vi "TSCAN_UDS.vi"(10 "Data":T3={"Communication message"={"Sender"="", "receiver"="", "message"="", "data"=variant}, "Data"={"Config_parameter"={"Bus_Type"=0, "Channel"=1, "Channels used"=1, "DLL_PATH"=path "", "Read message type"=1, "REC_Channel"=0}, "Send_parameter"={"SendData"=[0, 0, 0, 0, 0, 0, 0, 0, 0, 0, 0, 0, 0, 0, 0, 0, 0, 0, 0, 0, 0, 0, 0, 0, 0, 0, 0, 0, 0, 0, 0, 0, 0, 0, 0, 0, 0, 0, 0, 0, 0, 0, 0, 0, 0, 0, 0, 0, 0, 0, 0, 0, 0, 0, 0, 0, 0, 0, 0, 0, 0, 0, 0, 0, 0, 0, 0, 0, 0, 0, 0, 0, 0, 0, 0], "Data Length"=15, "ID"=0, "Frame Format"=0, "Frame Type"=0, "BRS"=enum."Close", "FD Frame"=0, "async&sync"=enum."async", "Timeout"=0}, "DBC_Ctr"={"DBC Path"=path "", "DBC loading channel"=0, "DatabaseId"=0, "DBMessages"=[], "DBSignals"=[]}, "CAN_Config_Array"=[], "CANFD_Config_Array"=[], "CAN_Config_Regs_Array"=[], "CANFD_Config_Regs_Array"=[], "Blf_Log"={"Blf_Log_PATH"=path ""}, "UDS"={"UDS Control"={"UDS Channel Index"=0, "Request ID"=1992, "Response ID"=2015, "Request ID (Func)"=1, "Session Mode"=1, "Reset Mode"=255, "DTC Mask"=0, "GropOfDTC"=0, "Seed Level"=2, "Seed"=[], "Key Level"=0, "Key"=[], "Read Identifier"=0, "UDS Read Data"=[], "ASCII Data"="", "Write Identifier"=0, "UDS Wrtie Data"=[], "IO Control Identifier"=1, "UDS IOControl Data"=[], "IO Control Mode"=0, "UDS IOControl Read Data"=[], "Routine Control Identifier"=0, "UDS RoutineControl Data"=[], "UDS RoutineControl Read Data"=[], "Routine Control Mode"=1, "SupportFDCAN"=TRUE, "time config"={"p2_timeout"=0, "p2_extended"=0, "s3_servertime"=0, "s3_clienttime"=0}, "ServiceLayer"={"FilledByte"=0, "STMin"=10, "BlockSize"=10, "FCDelay"=10, "MaxLength"=4095}, "Request"=[], "Respond"=[]}, "DiagModuleIndex"=1984}}, "CAN_Buffer"=[], "CANFD_Buffer"=[], "error in"={"status"=FALSE, "code"=0, "source"=""}, "CAN_Period_Datas"=[], "CANFD_period_Datas"=[], "CAN_Filtering_Datas"=[], "CANFD_Filtering_Datas"=[], "AsynCall?"=FALSE} {"Data"."UDS"."UDS Control"."Respond" format="%.0x"; "Data"."UDS"."UDS Control"."Request" format="%.0x"; "Data"."UDS"."UDS Control"."ServiceLayer"."FilledByte" format="%.0x"; "Data"."UDS"."UDS Control"."GropOfDTC" format="%.0x"; "Data"."UDS"."UDS Control"."DTC Mask" format="%.0x"; "Data"."UDS"."UDS Control"."UDS RoutineControl Read Data" format="%.0x"; "Data"."UDS"."UDS Control"."UDS RoutineControl Data" format="%.0x"; "Data"."UDS"."UDS Control"."Routine Control Identifier" format="%.0x"; "Data"."UDS"."UDS Control"."UDS IOControl Read Data" format="%.0x"; "Data"."UDS"."UDS Control"."UDS IOControl Data" format="%.0x"; "Data"."UDS"."UDS Control"."IO Control Identifier" format="%.0x"; "Data"."UDS"."UDS Control"."UDS Wrtie Data" format="%.0x"; "Data"."UDS"."UDS Control"."UDS Read Data" format="%.0x"; "Data"."UDS"."UDS Control"."Write Identifier" format="%.0x"; "Data"."UDS"."UDS Control"."Read Identifier" format="%.0x"; "Data"."UDS"."UDS Control"."Key" format="%.0x"; "Data"."UDS"."UDS Control"."Seed" format="%.0x"; "Data"."UDS"."UDS Control"."Request ID (Func)" format="%.0x"; "Data"."UDS"."UDS Control"."Response ID" format="%.0x"; "Data"."UDS"."UDS Control"."Request ID" format="%.0x"; "Data"."UDS"."UDS Control"."Session Mode" items=["DefaultSession"=1, "ProgrammingSession"=2, "ExtendedDiagnosticSession"=3]; "Data"."UDS"."UDS Control"."Reset Mode" items=["HardReset"=1, "keyOffOnReset"=2, "SoftReset"=3]; "Data"."UDS"."UDS Control"."IO Control Mode" items=["ReturnControlToECU", "ResetToDefault", "FreezeCurrentState", "ShortTermAdjustment"]; "Data"."UDS"."UDS Control"."Routine Control Mode" items=["Start routine"=1, "Stop routine"=2, "Request routine results"=3]; "Data"."CAN_Config_Regs_Array"."CAN configuration"."AAppChannel" items=["CHN1", "CHN2", "CHN3", "CHN4", "CHN5", "CHN6", "CHN7", "CHN8", "CHN9", "CHN10", "CHN11", "CHN12", "CHN13", "CHN14", "CHN15", "CHN16", "CHN17", "CHN18", "CHN19", "CHN20", "CHN21", "CHN22", "CHN23", "CHN24", "CHN25", "CHN26", "CHN27", "CHN28", "CHN29", "CHN30", "CHN31", "CHN32"]; "Data"."CAN_Config_Regs_Array"."CAN configuration"."AHwChannel" items=["CHN1", "CHN2", "CHN3", "CHN4", "CHN5", "CHN6", "CHN7", "CHN8", "CHN9", "CHN10", "CHN11", "CHN12", "CHN13", "CHN14", "CHN15", "CHN16", "CHN17", "CHN18", "CHN19", "CHN20", "CHN21", "CHN22", "CHN23", "CHN24", "CHN25", "CHN26", "CHN27", "CHN28", "CHN29", "CHN30", "CHN31", "CHN32"]; "Data"."CAN_Config_Regs_Array"."CAN configuration"."HardwareType" items=["BUS_UNKNOWN_TYPE", "TS_TCP_DEVICE", "XL_USB_DEVICE", "TS_USB_DEVICE", "PEAK_USB_DEVICE", "KVASER_USB_DEVICE", "ZLG_USB_DEVICE", "ICS_USB_DEVICE", "TS_TC1005_DEVICE", "CANABLE_USB_DEVICE", "TS_WIRELESS_OBD", "TS_USB_DEVICE_EX", "IXXAT_USB_DEVICE", "TS_ETH_IF_DEVICE", "TS_USB_IF_DEVICE", "BUS_DEV_TYPE_COUNT"]; "Data"."CANFD_Config_Regs_Array"."CANFD Configuration"."Hardware Type" items=["BUS_UNKNOWN_TYPE", "TS_TCP_DEVICE", "XL_USB_DEVICE", "TS_USB_DEVICE", "PEAK_USB_DEVICE", "KVASER_USB_DEVICE", "ZLG_USB_DEVICE", "ICS_USB_DEVICE", "TS_TC1005_DEVICE", "CANABLE_USB_DEVICE", "TS_WIRELESS_OBD", "TS_USB_DEVICE_EX", "IXXAT_USB_DEVICE", "TS_ETH_IF_DEVICE", "TS_USB_IF_DEVICE", "BUS_DEV_TYPE_COUNT"]; "Data"."CANFD_Config_Regs_Array"."CANFD Configuration"."AHwChannel" items=["CHN1", "CHN2", "CHN3", "CHN4", "CHN5", "CHN6", "CHN7", "CHN8", "CHN9", "CHN10", "CHN11", "CHN12", "CHN13", "CHN14", "CHN15", "CHN16", "CHN17", "CHN18", "CHN19", "CHN20", "CHN21", "CHN22", "CHN23", "CHN24", "CHN25", "CHN26", "CHN27", "CHN28", "CHN29", "CHN30", "CHN31", "CHN32"]; "Data"."CANFD_Config_Regs_Array"."CANFD Configuration"."AAppChannel" items=["CHN1", "CHN2", "CHN3", "CHN4", "CHN5", "CHN6", "CHN7", "CHN8", "CHN9", "CHN10", "CHN11", "CHN12", "CHN13", "CHN14", "CHN15", "CHN16", "CHN17", "CHN18", "CHN19", "CHN20", "CHN21", "CHN22", "CHN23", "CHN24", "CHN25", "CHN26", "CHN27", "CHN28", "CHN29", "CHN30", "CHN31", "CHN32"]; "Data"."CANFD_Config_Regs_Array"."CANFD Configuration"."AControllerType" items=["lfdtCAN", "lfdtISOFDCAN", "lfdtNonISOFDFDCAN"]; "Data"."CANFD_Config_Regs_Array"."CANFD Configuration"."AControllerMode" items=["lfdmNormal", "lfdmACKOff", "lfdmRestricted"]; "Data"."CANFD_Config_Array"."Hardware Type" items=["BUS_UNKNOWN_TYPE", "TS_TCP_DEVICE", "XL_USB_DEVICE", "TS_USB_DEVICE", "PEAK_USB_DEVICE", "KVASER_USB_DEVICE", "ZLG_USB_DEVICE", "ICS_USB_DEVICE", "TS_TC1005_DEVICE", "CANABLE_USB_DEVICE", "TS_WIRELESS_OBD", "TS_USB_DEVICE_EX", "IXXAT_USB_DEVICE", "TS_ETH_IF_DEVICE", "TS_USB_IF_DEVICE", "BUS_DEV_TYPE_COUNT"]; "Data"."CANFD_Config_Array"."AHwChannel" items=["CHN1", "CHN2", "CHN3", "CHN4", "CHN5", "CHN6", "CHN7", "CHN8", "CHN9", "CHN10", "CHN11", "CHN12", "CHN13", "CHN14", "CHN15", "CHN16", "CHN17", "CHN18", "CHN19", "CHN20", "CHN21", "CHN22", "CHN23", "CHN24", "CHN25", "CHN26", "CHN27", "CHN28", "CHN29", "CHN30", "CHN31", "CHN32"]; "Data"."CANFD_Config_Array"."AAppChannel" items=["CHN1", "CHN2", "CHN3", "CHN4", "CHN5", "CHN6", "CHN7", "CHN8", "CHN9", "CHN10", "CHN11", "CHN12", "CHN13", "CHN14", "CHN15", "CHN16", "CHN17", "CHN18", "CHN19", "CHN20", "CHN21", "CHN22", "CHN23", "CHN24", "CHN25", "CHN26", "CHN27", "CHN28", "CHN29", "CHN30", "CHN31", "CHN32"]; "Data"."CANFD_Config_Array"."AControllerType" items=["lfdtCAN", "lfdtISOFDCAN", "lfdtNonISOFDFDCAN"]; "Data"."CANFD_Config_Array"."AControllerMode" items=["lfdmNormal", "lfdmACKOff", "lfdmRestricted"]; "Data"."CAN_Config_Array"."AAppChannel" items=["CHN1", "CHN2", "CHN3", "CHN4", "CHN5", "CHN6", "CHN7", "CHN8", "CHN9", "CHN10", "CHN11", "CHN12", "CHN13", "CHN14", "CHN15", "CHN16", "CHN17", "CHN18", "CHN19", "CHN20", "CHN21", "CHN22", "CHN23", "CHN24", "CHN25", "CHN26", "CHN27", "CHN28", "CHN29", "CHN30", "CHN31", "CHN32"]; "Data"."CAN_Config_Array"."AHwChannel" items=["CHN1", "CHN2", "CHN3", "CHN4", "CHN5", "CHN6", "CHN7", "CHN8", "CHN9", "CHN10", "CHN11", "CHN12", "CHN13", "CHN14", "CHN15", "CHN16", "CHN17", "CHN18", "CHN19", "CHN20", "CHN21", "CHN22", "CHN23", "CHN24", "CHN25", "CHN26", "CHN27", "CHN28", "CHN29", "CHN30", "CHN31", "CHN32"]; "Data"."CAN_Config_Array"."HardwareType" items=["BUS_UNKNOWN_TYPE", "TS_TCP_DEVICE", "XL_USB_DEVICE", "TS_USB_DEVICE", "PEAK_USB_DEVICE", "KVASER_USB_DEVICE", "ZLG_USB_DEVICE", "ICS_USB_DEVICE", "TS_TC1005_DEVICE", "CANABLE_USB_DEVICE", "TS_WIRELESS_OBD", "TS_USB_DEVICE_EX", "IXXAT_USB_DEVICE", "TS_ETH_IF_DEVICE", "TS_USB_IF_DEVICE", "BUS_DEV_TYPE_COUNT"]; "Data"."DBC_Ctr"."DBSignals"."SignalList"."Message_Type" items=["CAN", "CANFD", "J1939"]; "Data"."DBC_Ctr"."DBSignals"."SignalList"."Mux_Type" items=["Normal", "multiplexor", "multiplexed"]; "Data"."DBC_Ctr"."DBSignals"."SignalList"."Is_Motorola" items=["Intel", "Motorola"]; "Data"."DBC_Ctr"."DBSignals"."SignalList"."Value_Type" items=["unsigned int", "signed int", "float", "double"]; "Data"."DBC_Ctr"."DBSignals"."SignalList"."ID" format="%.0x"; "Data"."DBC_Ctr"."DBMessages"."BRS" items=["No BRS", "BRS"]; "Data"."DBC_Ctr"."DBMessages"."ID" format="%.0x"; "Data"."DBC_Ctr"."DBMessages"."Type" items=["cftStdCAN", "cftExtCAN", "cftJ1939", "cftStdCANFD", "cftExtCANFD"]; "Data"."DBC_Ctr"."DBC loading channel" items=["CHN1", "CHN2", "CHN3", "CHN4", "CHN5", "CHN6", "CHN7", "CHN8", "CHN9", "CHN10", "CHN11", "CHN12", "CHN13", "CHN14", "CHN15", "CHN16", "CHN17", "CHN18", "CHN19", "CHN20", "CHN21", "CHN22", "CHN23", "CHN24", "CHN25", "CHN26", "CHN27", "CHN28", "CHN29", "CHN30", "CHN31", "CHN32"]; "Data"."Send_parameter"."FD Frame" items=["Ordinary CAN Data", "FD CAN Data"]; "Data"."Send_parameter"."Frame Type" items=["Standard Frame", "Extended Frame"]; "Data"."Send_parameter"."Frame Format" items=["Standard Frame", "Extended Frame"]; "Data"."Send_parameter"."ID" format="%x"; "Data"."Send_parameter"."Data Length" items=["0", "1", "2", "3", "4", "5", "6", "7", "8", "12", "16", "20", "24", "32", "48", "64"]; "Data"."Send_parameter"."SendData" format="%x"; "Data"."Config_parameter"."REC_Channel" items=["CHN1", "CHN2", "CHN3", "CHN4", "CHN5", "CHN6", "CHN7", "CHN8", "CHN9", "CHN10", "CHN11", "CHN12", "CHN13", "CHN14", "CHN15", "CHN16", "CHN17", "CHN18", "CHN19", "CHN20", "CHN21", "CHN22", "CHN23", "CHN24", "CHN25", "CHN26", "CHN27", "CHN28", "CHN29", "CHN30", "CHN31", "CHN32"]; "Data"."Config_parameter"."Read message type" items=["Only read received messages", "Receive&send messages"]; "Data"."Config_parameter"."Channels used" items=["1 Channel"=1, "2 Channels"=2, "3 Channels"=3, "4 Channels"=4, "5 Channels"=5, "6 Channels"=6, "7 Channels"=7, "8 Channels"=8, "9 Channels"=9, "10 Channels"=10, "11 Channels"=11, "12 Channels"=12, "13 Channels"=13, "14 Channels"=14, "15 Channels"=15, "16 Channels"=16]; "Data"."Config_parameter"."Channel" items=["Disable", "Enable"]; "Data"."Config_parameter"."Bus_Type" items=["CAN", "CANFD"]}, 11 "Sender":string="Demo") -> (2 "Data out":T3={"Communication message"={"Sender"="", "receiver"="", "message"="", "data"=variant}, "Data"={"Config_parameter"={"Bus_Type"=0, "Channel"=1, "Channels used"=1, "DLL_PATH"=path "", "Read message type"=1, "REC_Channel"=0}, "Send_parameter"={"SendData"=[0, 0, 0, 0, 0, 0, 0, 0, 0, 0, 0, 0, 0, 0, 0, 0, 0, 0, 0, 0, 0, 0, 0, 0, 0, 0, 0, 0, 0, 0, 0, 0, 0, 0, 0, 0, 0, 0, 0, 0, 0, 0, 0, 0, 0, 0, 0, 0, 0, 0, 0, 0, 0, 0, 0, 0, 0, 0, 0, 0, 0, 0, 0, 0, 0, 0, 0, 0, 0, 0, 0, 0, 0, 0, 0], "Data Length"=15, "ID"=0, "Frame Format"=0, "Frame Type"=0, "BRS"=enum."Close", "FD Frame"=0, "async&sync"=enum."async", "Timeout"=0}, "DBC_Ctr"={"DBC Path"=path "", "DBC loading channel"=0, "DatabaseId"=0, "DBMessages"=[], "DBSignals"=[]}, "CAN_Config_Array"=[], "CANFD_Config_Array"=[], "CAN_Config_Regs_Array"=[], "CANFD_Config_Regs_Array"=[], "Blf_Log"={"Blf_Log_PATH"=path ""}, "UDS"={"UDS Control"={"UDS Channel Index"=0, "Request ID"=1992, "Response ID"=2015, "Request ID (Func)"=1, "Session Mode"=1, "Reset Mode"=255, "DTC Mask"=0, "GropOfDTC"=0, "Seed Level"=2, "Seed"=[], "Key Level"=0, "Key"=[], "Read Identifier"=0, "UDS Read Data"=[], "ASCII Data"="", "Write Identifier"=0, "UDS Wrtie Data"=[], "IO Control Identifier"=1, "UDS IOControl Data"=[], "IO Control Mode"=0, "UDS IOControl Read Data"=[], "Routine Control Identifier"=0, "UDS RoutineControl Data"=[], "UDS RoutineControl Read Data"=[], "Routine Control Mode"=1, "SupportFDCAN"=TRUE, "time config"={"p2_timeout"=0, "p2_extended"=0, "s3_servertime"=0, "s3_clienttime"=0}, "ServiceLayer"={"FilledByte"=0, "STMin"=10, "BlockSize"=10, "FCDelay"=10, "MaxLength"=4095}, "Request"=[], "Respond"=[]}, "DiagModuleIndex"=1984}}, "CAN_Buffer"=[], "CANFD_Buffer"=[], "error in"={"status"=FALSE, "code"=0, "source"=""}, "CAN_Period_Datas"=[], "CANFD_period_Datas"=[], "CAN_Filtering_Datas"=[], "CANFD_Filtering_Datas"=[], "AsynCall?"=FALSE} {"Data"."UDS"."UDS Control"."Respond" format="%.0x"; "Data"."UDS"."UDS Control"."Request" format="%.0x"; "Data"."UDS"."UDS Control"."ServiceLayer"."FilledByte" format="%.0x"; "Data"."UDS"."UDS Control"."GropOfDTC" format="%.0x"; "Data"."UDS"."UDS Control"."DTC Mask" format="%.0x"; "Data"."UDS"."UDS Control"."UDS RoutineControl Read Data" format="%.0x"; "Data"."UDS"."UDS Control"."UDS RoutineControl Data" format="%.0x"; "Data"."UDS"."UDS Control"."Routine Control Identifier" format="%.0x"; "Data"."UDS"."UDS Control"."UDS IOControl Read Data" format="%.0x"; "Data"."UDS"."UDS Control"."UDS IOControl Data" format="%.0x"; "Data"."UDS"."UDS Control"."IO Control Identifier" format="%.0x"; "Data"."UDS"."UDS Control"."UDS Wrtie Data" format="%.0x"; "Data"."UDS"."UDS Control"."UDS Read Data" format="%.0x"; "Data"."UDS"."UDS Control"."Write Identifier" format="%.0x"; "Data"."UDS"."UDS Control"."Read Identifier" format="%.0x"; "Data"."UDS"."UDS Control"."Key" format="%.0x"; "Data"."UDS"."UDS Control"."Seed" format="%.0x"; "Data"."UDS"."UDS Control"."Request ID (Func)" format="%.0x"; "Data"."UDS"."UDS Control"."Response ID" format="%.0x"; "Data"."UDS"."UDS Control"."Request ID" format="%.0x"; "Data"."UDS"."UDS Control"."Session Mode" items=["DefaultSession"=1, "ProgrammingSession"=2, "ExtendedDiagnosticSession"=3]; "Data"."UDS"."UDS Control"."Reset Mode" items=["HardReset"=1, "keyOffOnReset"=2, "SoftReset"=3]; "Data"."UDS"."UDS Control"."IO Control Mode" items=["ReturnControlToECU", "ResetToDefault", "FreezeCurrentState", "ShortTermAdjustment"]; "Data"."UDS"."UDS Control"."Routine Control Mode" items=["Start routine"=1, "Stop routine"=2, "Request routine results"=3]; "Data"."CAN_Config_Regs_Array"."CAN configuration"."AAppChannel" items=["CHN1", "CHN2", "CHN3", "CHN4", "CHN5", "CHN6", "CHN7", "CHN8", "CHN9", "CHN10", "CHN11", "CHN12", "CHN13", "CHN14", "CHN15", "CHN16", "CHN17", "CHN18", "CHN19", "CHN20", "CHN21", "CHN22", "CHN23", "CHN24", "CHN25", "CHN26", "CHN27", "CHN28", "CHN29", "CHN30", "CHN31", "CHN32"]; "Data"."CAN_Config_Regs_Array"."CAN configuration"."AHwChannel" items=["CHN1", "CHN2", "CHN3", "CHN4", "CHN5", "CHN6", "CHN7", "CHN8", "CHN9", "CHN10", "CHN11", "CHN12", "CHN13", "CHN14", "CHN15", "CHN16", "CHN17", "CHN18", "CHN19", "CHN20", "CHN21", "CHN22", "CHN23", "CHN24", "CHN25", "CHN26", "CHN27", "CHN28", "CHN29", "CHN30", "CHN31", "CHN32"]; "Data"."CAN_Config_Regs_Array"."CAN configuration"."HardwareType" items=["BUS_UNKNOWN_TYPE", "TS_TCP_DEVICE", "XL_USB_DEVICE", "TS_USB_DEVICE", "PEAK_USB_DEVICE", "KVASER_USB_DEVICE", "ZLG_USB_DEVICE", "ICS_USB_DEVICE", "TS_TC1005_DEVICE", "CANABLE_USB_DEVICE", "TS_WIRELESS_OBD", "TS_USB_DEVICE_EX", "IXXAT_USB_DEVICE", "TS_ETH_IF_DEVICE", "TS_USB_IF_DEVICE", "BUS_DEV_TYPE_COUNT"]; "Data"."CANFD_Config_Regs_Array"."CANFD Configuration"."Hardware Type" items=["BUS_UNKNOWN_TYPE", "TS_TCP_DEVICE", "XL_USB_DEVICE", "TS_USB_DEVICE", "PEAK_USB_DEVICE", "KVASER_USB_DEVICE", "ZLG_USB_DEVICE", "ICS_USB_DEVICE", "TS_TC1005_DEVICE", "CANABLE_USB_DEVICE", "TS_WIRELESS_OBD", "TS_USB_DEVICE_EX", "IXXAT_USB_DEVICE", "TS_ETH_IF_DEVICE", "TS_USB_IF_DEVICE", "BUS_DEV_TYPE_COUNT"]; "Data"."CANFD_Config_Regs_Array"."CANFD Configuration"."AHwChannel" items=["CHN1", "CHN2", "CHN3", "CHN4", "CHN5", "CHN6", "CHN7", "CHN8", "CHN9", "CHN10", "CHN11", "CHN12", "CHN13", "CHN14", "CHN15", "CHN16", "CHN17", "CHN18", "CHN19", "CHN20", "CHN21", "CHN22", "CHN23", "CHN24", "CHN25", "CHN26", "CHN27", "CHN28", "CHN29", "CHN30", "CHN31", "CHN32"]; "Data"."CANFD_Config_Regs_Array"."CANFD Configuration"."AAppChannel" items=["CHN1", "CHN2", "CHN3", "CHN4", "CHN5", "CHN6", "CHN7", "CHN8", "CHN9", "CHN10", "CHN11", "CHN12", "CHN13", "CHN14", "CHN15", "CHN16", "CHN17", "CHN18", "CHN19", "CHN20", "CHN21", "CHN22", "CHN23", "CHN24", "CHN25", "CHN26", "CHN27", "CHN28", "CHN29", "CHN30", "CHN31", "CHN32"]; "Data"."CANFD_Config_Regs_Array"."CANFD Configuration"."AControllerType" items=["lfdtCAN", "lfdtISOFDCAN", "lfdtNonISOFDFDCAN"]; "Data"."CANFD_Config_Regs_Array"."CANFD Configuration"."AControllerMode" items=["lfdmNormal", "lfdmACKOff", "lfdmRestricted"]; "Data"."CANFD_Config_Array"."Hardware Type" items=["BUS_UNKNOWN_TYPE", "TS_TCP_DEVICE", "XL_USB_DEVICE", "TS_USB_DEVICE", "PEAK_USB_DEVICE", "KVASER_USB_DEVICE", "ZLG_USB_DEVICE", "ICS_USB_DEVICE", "TS_TC1005_DEVICE", "CANABLE_USB_DEVICE", "TS_WIRELESS_OBD", "TS_USB_DEVICE_EX", "IXXAT_USB_DEVICE", "TS_ETH_IF_DEVICE", "TS_USB_IF_DEVICE", "BUS_DEV_TYPE_COUNT"]; "Data"."CANFD_Config_Array"."AHwChannel" items=["CHN1", "CHN2", "CHN3", "CHN4", "CHN5", "CHN6", "CHN7", "CHN8", "CHN9", "CHN10", "CHN11", "CHN12", "CHN13", "CHN14", "CHN15", "CHN16", "CHN17", "CHN18", "CHN19", "CHN20", "CHN21", "CHN22", "CHN23", "CHN24", "CHN25", "CHN26", "CHN27", "CHN28", "CHN29", "CHN30", "CHN31", "CHN32"]; "Data"."CANFD_Config_Array"."AAppChannel" items=["CHN1", "CHN2", "CHN3", "CHN4", "CHN5", "CHN6", "CHN7", "CHN8", "CHN9", "CHN10", "CHN11", "CHN12", "CHN13", "CHN14", "CHN15", "CHN16", "CHN17", "CHN18", "CHN19", "CHN20", "CHN21", "CHN22", "CHN23", "CHN24", "CHN25", "CHN26", "CHN27", "CHN28", "CHN29", "CHN30", "CHN31", "CHN32"]; "Data"."CANFD_Config_Array"."AControllerType" items=["lfdtCAN", "lfdtISOFDCAN", "lfdtNonISOFDFDCAN"]; "Data"."CANFD_Config_Array"."AControllerMode" items=["lfdmNormal", "lfdmACKOff", "lfdmRestricted"]; "Data"."CAN_Config_Array"."AAppChannel" items=["CHN1", "CHN2", "CHN3", "CHN4", "CHN5", "CHN6", "CHN7", "CHN8", "CHN9", "CHN10", "CHN11", "CHN12", "CHN13", "CHN14", "CHN15", "CHN16", "CHN17", "CHN18", "CHN19", "CHN20", "CHN21", "CHN22", "CHN23", "CHN24", "CHN25", "CHN26", "CHN27", "CHN28", "CHN29", "CHN30", "CHN31", "CHN32"]; "Data"."CAN_Config_Array"."AHwChannel" items=["CHN1", "CHN2", "CHN3", "CHN4", "CHN5", "CHN6", "CHN7", "CHN8", "CHN9", "CHN10", "CHN11", "CHN12", "CHN13", "CHN14", "CHN15", "CHN16", "CHN17", "CHN18", "CHN19", "CHN20", "CHN21", "CHN22", "CHN23", "CHN24", "CHN25", "CHN26", "CHN27", "CHN28", "CHN29", "CHN30", "CHN31", "CHN32"]; "Data"."CAN_Config_Array"."HardwareType" items=["BUS_UNKNOWN_TYPE", "TS_TCP_DEVICE", "XL_USB_DEVICE", "TS_USB_DEVICE", "PEAK_USB_DEVICE", "KVASER_USB_DEVICE", "ZLG_USB_DEVICE", "ICS_USB_DEVICE", "TS_TC1005_DEVICE", "CANABLE_USB_DEVICE", "TS_WIRELESS_OBD", "TS_USB_DEVICE_EX", "IXXAT_USB_DEVICE", "TS_ETH_IF_DEVICE", "TS_USB_IF_DEVICE", "BUS_DEV_TYPE_COUNT"]; "Data"."DBC_Ctr"."DBSignals"."SignalList"."Message_Type" items=["CAN", "CANFD", "J1939"]; "Data"."DBC_Ctr"."DBSignals"."SignalList"."Mux_Type" items=["Normal", "multiplexor", "multiplexed"]; "Data"."DBC_Ctr"."DBSignals"."SignalList"."Is_Motorola" items=["Intel", "Motorola"]; "Data"."DBC_Ctr"."DBSignals"."SignalList"."Value_Type" items=["unsigned int", "signed int", "float", "double"]; "Data"."DBC_Ctr"."DBSignals"."SignalList"."ID" format="%.0x"; "Data"."DBC_Ctr"."DBMessages"."BRS" items=["No BRS", "BRS"]; "Data"."DBC_Ctr"."DBMessages"."ID" format="%.0x"; "Data"."DBC_Ctr"."DBMessages"."Type" items=["cftStdCAN", "cftExtCAN", "cftJ1939", "cftStdCANFD", "cftExtCANFD"]; "Data"."DBC_Ctr"."DBC loading channel" items=["CHN1", "CHN2", "CHN3", "CHN4", "CHN5", "CHN6", "CHN7", "CHN8", "CHN9", "CHN10", "CHN11", "CHN12", "CHN13", "CHN14", "CHN15", "CHN16", "CHN17", "CHN18", "CHN19", "CHN20", "CHN21", "CHN22", "CHN23", "CHN24", "CHN25", "CHN26", "CHN27", "CHN28", "CHN29", "CHN30", "CHN31", "CHN32"]; "Data"."Send_parameter"."FD Frame" items=["Ordinary CAN Data", "FD CAN Data"]; "Data"."Send_parameter"."Frame Type" items=["Standard Frame", "Extended Frame"]; "Data"."Send_parameter"."Frame Format" items=["Standard Frame", "Extended Frame"]; "Data"."Send_parameter"."ID" format="%x"; "Data"."Send_parameter"."Data Length" items=["0", "1", "2", "3", "4", "5", "6", "7", "8", "12", "16", "20", "24", "32", "48", "64"]; "Data"."Send_parameter"."SendData" format="%x"; "Data"."Config_parameter"."REC_Channel" items=["CHN1", "CHN2", "CHN3", "CHN4", "CHN5", "CHN6", "CHN7", "CHN8", "CHN9", "CHN10", "CHN11", "CHN12", "CHN13", "CHN14", "CHN15", "CHN16", "CHN17", "CHN18", "CHN19", "CHN20", "CHN21", "CHN22", "CHN23", "CHN24", "CHN25", "CHN26", "CHN27", "CHN28", "CHN29", "CHN30", "CHN31", "CHN32"]; "Data"."Config_parameter"."Read message type" items=["Only read received messages", "Receive&send messages"]; "Data"."Config_parameter"."Channels used" items=["1 Channel"=1, "2 Channels"=2, "3 Channels"=3, "4 Channels"=4, "5 Channels"=5, "6 Channels"=6, "7 Channels"=7, "8 Channels"=8, "9 Channels"=9, "10 Channels"=10, "11 Channels"=11, "12 Channels"=12, "13 Channels"=13, "14 Channels"=14, "15 Channels"=15, "16 Channels"=16]; "Data"."Config_parameter"."Channel" items=["Disable", "Enable"]; "Data"."Config_parameter"."Bus_Type" items=["CAN", "CANFD"]})   [LabVIEW 2014]
uses:
  <vilib>/Utility/miscctls.llb/LVPointTypeDef.ctl
  Diagnosis/Typedef/UDS Control.ctl
  Diagnosis/Typedef/UDS Cluster.ctl
  Typedef/TSCAN_Config_parameter.ctl
  Typedef/TSCAN_Send_parameter.ctl
  DataBase/Typedef/DBMessage.ctl
  DataBase/Typedef/DBSignal.ctl
  Typedef/TSCAN_DBC_Ctr.ctl
  All_Control/Typedef/Hardware Type.ctl
  Utilities/Typedef/Hardware_Subtype.ctl
  Typedef/TSCAN_CAN_Configuration.ctl
  Typedef/TSCAN_CANFD_Configuration.ctl
  Typedef/TSCAN_CANFD_Configuration_Regs.ctl
  Typedef/TSCAN_CAN_Configuration_Regs.ctl
  All_Control/Typedef/Blf_Log.ctl
  Typedef/TSCAN_CAN_CANFD_Demo_Data.ctl
  Typedef/TSCAN_CAN_CANFD_Demo_Data1.ctl
panel:
  out "pDiagModuleIndex":i32
  out "Size":u32
  out "Respond":u8[](array[numeric]) format="%.0x"
  in  "UDS Execute":bool
  in  "Request":u8[](array[numeric]) format="%.0x"
  in  "ServiceLayer":T1={"FilledByte"=0, "STMin"=10, "BlockSize"=10, "FCDelay"=10, "MaxLength"=4095} {"FilledByte" format="%.0x"}
  in  "ServiceLayer_setting":bool
  in  "time config setting":bool
  in  "time config":T2
  out "Create Session successful":bool
  in  "UDS RoutineControl Read Data":u8[](array[numeric]) caption="Data" format="%.0x"
  in  "Routine Control Mode":u8(ring)=1 caption="Mode" items=["Start routine"=1, "Stop routine"=2, "Request routine results"=3]
  in  "UDS RoutineControl Data":u8[](array[numeric]) caption="Data" format="%.0x"
  in  "Routine Control Identifier":u16 caption="Identifier" format="%.0x"
  in  "UDS RoutineControl by Identifier":bool
  in  "UDS IOControl Read Data":u8[](array[numeric]) caption="Data" format="%.0x"
  in  "IO Control Mode":u8(ring) caption="Mode" items=["ReturnControlToECU", "ResetToDefault", "FreezeCurrentState", "ShortTermAdjustment"]
  in  "UDS IOControl Data":u8[](array[numeric]) caption="Data" format="%.0x"
  in  "IO Control Identifier":u16 caption="Identifier" format="%.0x"
  in  "UDS IOControl by Identifier":bool
  in  "UDS Wrtie Data":u8[](array[numeric]) caption="Data" format="%.0x"
  in  "Write Identifier":u16 caption="Identifier" format="%.0x"
  in  "UDS Write by Identifier":bool
  in  "ASCII Data":string
  in  "UDS Read Data":u8[](array[numeric]) caption="Data" format="%.0x"
  in  "Read Identifier":u16 caption="Identifier" format="%.0x"
  in  "UDS Read by Identifier":bool
  in  "Key":u8[](array[numeric]) format="%.0x"
  in  "Key Level":i32=2
  in  "UDS Send Key":bool
  in  "Seed":u8[](array[numeric]) format="%.0x"
  in  "Seed Level":i32=1
  in  "UDS Request Seed":bool
  in  "GropOfDTC":u32=16777215 format="%.0x"
  in  "UDS Clear DTC":bool
  in  "DTC Mask":u8=255 format="%.0x"
  in  "UDS Read DTC":bool
  in  "UDS TestPresent":bool
  in  "Reset Mode":u8(ring)=1 items=["HardReset"=1, "keyOffOnReset"=2, "SoftReset"=3]
  in  "UDS ECU Reset":bool
  in  "Session Mode":u8(ring)=1 items=["DefaultSession"=1, "ProgrammingSession"=2, "ExtendedDiagnosticSession"=3]
  in  "UDS Session Control":bool
  in  "UDS Delete Session":bool
  in  "UDS Create Session":bool
  in  "SupportFDCAN":bool=TRUE
  in  "UDS Channel Index":u32 caption="Channel Index"
  in  "Request ID (Func)":u32 format="%.0x"
  in  "Response ID":u32 format="%.0x"
  in  "Request ID":u32 format="%.0x"
  in  "log":i32(listbox)
  in  "Quit":bool
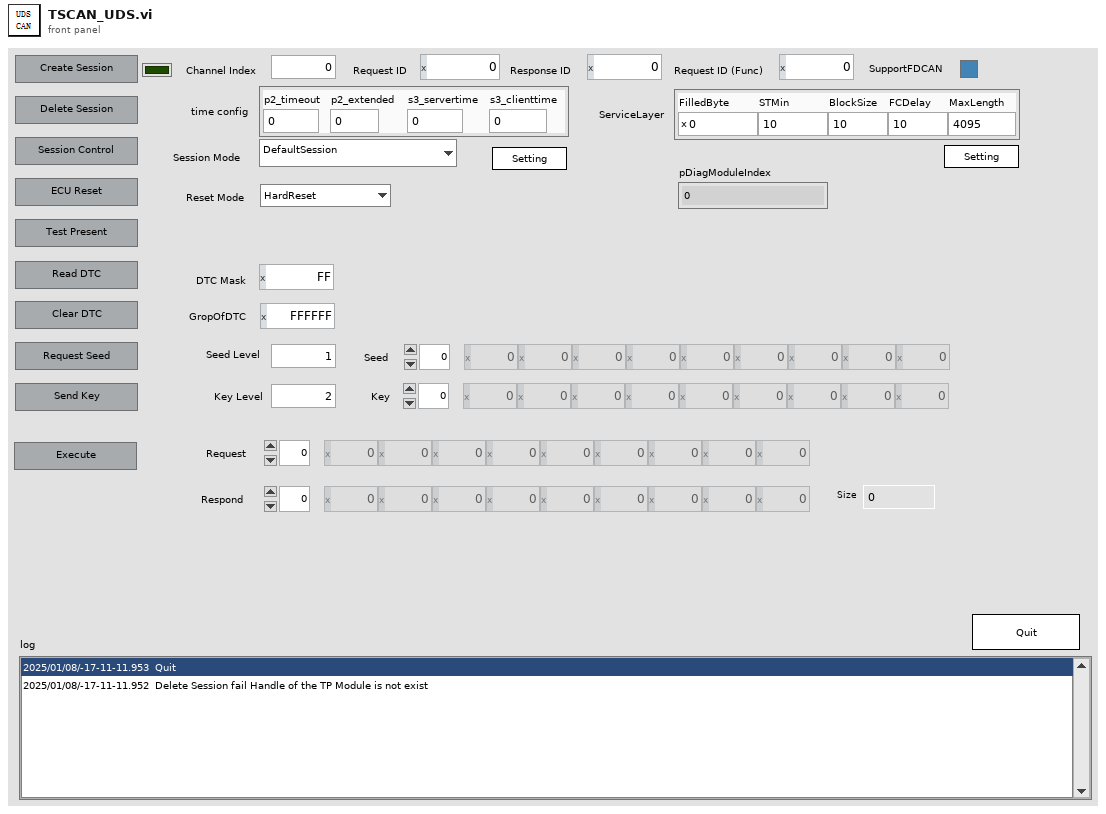
[diagram p1: front panel]
types:
  T1 = cluster{"FilledByte":u8, "STMin":i32, "BlockSize":i32, "FCDelay":i32, "MaxLength":i32}
  T2 = cluster{"p2_timeout":i32, "p2_extended":i32, "s3_servertime":i32, "s3_clienttime":i32}
  T3 = typedef "TSCAN_CAN_CANFD_Demo_Data1.ctl" = cluster{"Communication message":cluster{"Sender":string, "receiver":string, "message":string, "data":variant}, "Data":T4, "CAN_Buffer":cluster{"FIdxChn":u8, "FProperties":u8, "FDLC":u8, "FReserved":u8, "FIdentifier":i32, "FTimeUS":u64, "FData":cluster{"Data0":u8, "Data1":u8, "Data2":u8, "Data3":u8, "Data4":u8, "Data5":u8, "Data6":u8, "Data7":u8}}[], "CANFD_Buffer":cluster{"FIdxChn":u8, "FProperties":u8, "FDLC":u8, "FReserved":u8, "FIdentifier":i32, "FTimeUS":u64, "FDatas":cluster{"Initialize array[0]":u8, "Initialize array[1]":u8, "Initialize array[2]":u8, "Initialize array[3]":u8, "Initialize array[4]":u8, "Initialize array[5]":u8, "Initialize array[6]":u8, "Initialize array[7]":u8, "Initialize array[8]":u8, "Initialize array[9]":u8, "Initialize array[10]":u8, "Initialize array[11]":u8, "Initialize array[12]":u8, "Initialize array[13]":u8, "Initialize array[14]":u8, "Initialize array[15]":u8, "Initialize array[16]":u8, "Initialize array[17]":u8, "Initialize array[18]":u8, "Initialize array[19]":u8, "Initialize array[20]":u8, "Initialize array[21]":u8, "Initialize array[22]":u8, "Initialize array[23]":u8, "Initialize array[24]":u8, "Initialize array[25]":u8, "Initialize array[26]":u8, "Initialize array[27]":u8, "Initialize array[28]":u8, "Initialize array[29]":u8, "Initialize array[30]":u8, "Initialize array[31]":u8, "Initialize array[32]":u8, "Initialize array[33]":u8, "Initialize array[34]":u8, "Initialize array[35]":u8, "Initialize array[36]":u8, "Initialize array[37]":u8, "Initialize array[38]":u8, "Initialize array[39]":u8, "Initialize array[40]":u8, "Initialize array[41]":u8, "Initialize array[42]":u8, "Initialize array[43]":u8, "Initialize array[44]":u8, "Initialize array[45]":u8, "Initialize array[46]":u8, "Initialize array[47]":u8, "Initialize array[48]":u8, "Initialize array[49]":u8, "Initialize array[50]":u8, "Initialize array[51]":u8, "Initialize array[52]":u8, "Initialize array[53]":u8, "Initialize array[54]":u8, "Initialize array[55]":u8, "Initialize array[56]":u8, "Initialize array[57]":u8, "Initialize array[58]":u8, "Initialize array[59]":u8, "Initialize array[60]":u8, "Initialize array[61]":u8, "Initialize array[62]":u8, "Initialize array[63]":u8}}[], "error in":errorcluster, "CAN_Period_Datas":cluster{"FIdxChn":u8, "FProperties":u8, "FDLC":u8, "FReserved":u8, "FIdentifier":i32, "FTimeUS":u64, "FData":cluster{"Data0":u8, "Data1":u8, "Data2":u8, "Data3":u8, "Data4":u8, "Data5":u8, "Data6":u8, "Data7":u8}}[], "CANFD_period_Datas":cluster{"FIdxChn":u8, "FProperties":u8, "FDLC":u8, "FReserved":u8, "FIdentifier":i32, "FTimeUS":u64, "FDatas":cluster{"Initialize array[0]":u8, "Initialize array[1]":u8, "Initialize array[2]":u8, "Initialize array[3]":u8, "Initialize array[4]":u8, "Initialize array[5]":u8, "Initialize array[6]":u8, "Initialize array[7]":u8, "Initialize array[8]":u8, "Initialize array[9]":u8, "Initialize array[10]":u8, "Initialize array[11]":u8, "Initialize array[12]":u8, "Initialize array[13]":u8, "Initialize array[14]":u8, "Initialize array[15]":u8, "Initialize array[16]":u8, "Initialize array[17]":u8, "Initialize array[18]":u8, "Initialize array[19]":u8, "Initialize array[20]":u8, "Initialize array[21]":u8, "Initialize array[22]":u8, "Initialize array[23]":u8, "Initialize array[24]":u8, "Initialize array[25]":u8, "Initialize array[26]":u8, "Initialize array[27]":u8, "Initialize array[28]":u8, "Initialize array[29]":u8, "Initialize array[30]":u8, "Initialize array[31]":u8, "Initialize array[32]":u8, "Initialize array[33]":u8, "Initialize array[34]":u8, "Initialize array[35]":u8, "Initialize array[36]":u8, "Initialize array[37]":u8, "Initialize array[38]":u8, "Initialize array[39]":u8, "Initialize array[40]":u8, "Initialize array[41]":u8, "Initialize array[42]":u8, "Initialize array[43]":u8, "Initialize array[44]":u8, "Initialize array[45]":u8, "Initialize array[46]":u8, "Initialize array[47]":u8, "Initialize array[48]":u8, "Initialize array[49]":u8, "Initialize array[50]":u8, "Initialize array[51]":u8, "Initialize array[52]":u8, "Initialize array[53]":u8, "Initialize array[54]":u8, "Initialize array[55]":u8, "Initialize array[56]":u8, "Initialize array[57]":u8, "Initialize array[58]":u8, "Initialize array[59]":u8, "Initialize array[60]":u8, "Initialize array[61]":u8, "Initialize array[62]":u8, "Initialize array[63]":u8}}[], "CAN_Filtering_Datas":cluster{"FIdxChn":u8, "FProperties":u8, "FDLC":u8, "FReserved":u8, "FIdentifier":i32, "FTimeUS":u64, "FData":cluster{"Data0":u8, "Data1":u8, "Data2":u8, "Data3":u8, "Data4":u8, "Data5":u8, "Data6":u8, "Data7":u8}}[], "CANFD_Filtering_Datas":cluster{"FIdxChn":u8, "FProperties":u8, "FDLC":u8, "FReserved":u8, "FIdentifier":i32, "FTimeUS":u64, "FDatas":cluster{"Initialize array[0]":u8, "Initialize array[1]":u8, "Initialize array[2]":u8, "Initialize array[3]":u8, "Initialize array[4]":u8, "Initialize array[5]":u8, "Initialize array[6]":u8, "Initialize array[7]":u8, "Initialize array[8]":u8, "Initialize array[9]":u8, "Initialize array[10]":u8, "Initialize array[11]":u8, "Initialize array[12]":u8, "Initialize array[13]":u8, "Initialize array[14]":u8, "Initialize array[15]":u8, "Initialize array[16]":u8, "Initialize array[17]":u8, "Initialize array[18]":u8, "Initialize array[19]":u8, "Initialize array[20]":u8, "Initialize array[21]":u8, "Initialize array[22]":u8, "Initialize array[23]":u8, "Initialize array[24]":u8, "Initialize array[25]":u8, "Initialize array[26]":u8, "Initialize array[27]":u8, "Initialize array[28]":u8, "Initialize array[29]":u8, "Initialize array[30]":u8, "Initialize array[31]":u8, "Initialize array[32]":u8, "Initialize array[33]":u8, "Initialize array[34]":u8, "Initialize array[35]":u8, "Initialize array[36]":u8, "Initialize array[37]":u8, "Initialize array[38]":u8, "Initialize array[39]":u8, "Initialize array[40]":u8, "Initialize array[41]":u8, "Initialize array[42]":u8, "Initialize array[43]":u8, "Initialize array[44]":u8, "Initialize array[45]":u8, "Initialize array[46]":u8, "Initialize array[47]":u8, "Initialize array[48]":u8, "Initialize array[49]":u8, "Initialize array[50]":u8, "Initialize array[51]":u8, "Initialize array[52]":u8, "Initialize array[53]":u8, "Initialize array[54]":u8, "Initialize array[55]":u8, "Initialize array[56]":u8, "Initialize array[57]":u8, "Initialize array[58]":u8, "Initialize array[59]":u8, "Initialize array[60]":u8, "Initialize array[61]":u8, "Initialize array[62]":u8, "Initialize array[63]":u8}}[], "AsynCall?":bool}
  T4 = typedef "TSCAN_CAN_CANFD_Demo_Data.ctl" = cluster{"Config_parameter":T5, "Send_parameter":T6, "DBC_Ctr":T7, "CAN_Config_Array":T10[], "CANFD_Config_Array":T13[], "CAN_Config_Regs_Array":T14[], "CANFD_Config_Regs_Array":T15[], "Blf_Log":T16, "UDS":T17}
  T5 = typedef "TSCAN_Config_parameter.ctl" = cluster{"Bus_Type":u16, "Channel":i32, "Channels used":u16, "DLL_PATH":path, "Read message type":u16, "REC_Channel":i32}
  T6 = typedef "TSCAN_Send_parameter.ctl" = cluster{"SendData":u8[], "Data Length":i32, "ID":i32, "Frame Format":u8, "Frame Type":u8, "BRS":enum16{"Close", "Open"}, "FD Frame":u8, "async&sync":enum16{"async", "sync"}, "Timeout":u16}
  T7 = typedef "TSCAN_DBC_Ctr.ctl" = cluster{"DBC Path":path, "DBC loading channel":i32, "DatabaseId":u32, "DBMessages":T8[], "DBSignals":cluster{"MessageName":string, "SignalList":T9[]}[]}
  T8 = typedef "DBMessage.ctl" = cluster{"Type":u16, "DLC":i32, "ID":i32, "CycleTime":dbl, "Name":string, "Comment":string, "TX_Node_Index":i32, "Owned_Signal_List_Count ":i32, "Owned_Signal_List_Signal_Index":i32, "BRS":i32}
  T9 = typedef "DBSignal.ctl" = cluster{"ID":i32, "Value_Type":i32, "Is_Motorola":i32, "ValTab_Index":i32, "Mux_Type":i32, "Mux_Value":dbl, "Layout_Start":i32, "Length":i32, "Factor":dbl, "Offset":dbl, "InitValue":dbl, "Min":dbl, "Max":dbl, "Name":string, "Unit":string, "Comment":string, "Message_Index":i32, "Message_Type":i32}
  T10 = typedef "TSCAN_CAN_Configuration.ctl" = cluster{"HardwareType":T11, "Hardware Subtype":T12, "ABaudrateKbps":sgl, "AListenOnly":enum16{"Normal", "ListenOnly"}, "Int120Ohm":enum16{"Disable", "Enable"}, "EnableChannel":enum16{"Disable", "Enable"}, "AHwChannel":i32, "AAppChannel":i32, "AldHW":i32}
  T11 = typedef "Hardware Type.ctl" = i32
  T12 = typedef "Hardware_Subtype.ctl" = enum16{"TS_UNKNOWN_DEVICE", "TSCAN_PRO", "TSCAN_Lite1", "TC1001", "TL1001", "TC1011", "TM5011", "TC1002", "TC1014", "TSCANFD2517", "TC1026", "TC1016", "TC1012", "TC1013", "TLog1002", "TC1034", "TC1018", "GW2116", "TC2115", "MP1013", "TC1113", "TC1114", "TP1013", "TC1017", "TP1018", "TF10XX", "TL1004_FD_4_LIN_2", "TE1051", "TP1051", "TP1034", "TTS9015", "TP1026", "TTS1026", "TTS1034", "TTS1018", "TL1011", "TTS1015_LiAuto", "TTS1013_LiAuto", "TTS1016Pro", "TC1054Pro", "TC1054", "TLog1038", "TO1013", "TC1034Pro", "TC1018Pro", "TC1038Pro", "TS_DEV_END"}
  T13 = typedef "TSCAN_CANFD_Configuration.ctl" = cluster{"Hardware Type":T11, "Hardware Subtype":T12, "AArbRateKbps":sgl, "AListenOnly":enum16{"Normal", "ListenOnly"}, "Int120Ohm":enum16{"Disable", "Enable"}, "EnableChannel":enum16{"Disable", "Enable"}, "AHwChannel":i32, "AAppChannel":i32, "ADataRateKbps":sgl, "AControllerType":i32, "AControllerMode":i32, "AldHW":i32}
  T14 = typedef "TSCAN_CAN_Configuration_Regs.ctl" = cluster{"CAN_Sampling point":cluster{"ASEG1":i32, "ASEG2":i32, "APrescaler":i32, "ASJW":i32}, "CAN configuration":T10}
  T15 = typedef "TSCAN_CANFD_Configuration_Regs.ctl" = cluster{"CANFD Configuration":T13, "CANFD_Sampling point":cluster{"AArbSEG1":i32, "AArbSEG2":i32, "AArbPrescaler":i32, "AArbSJW":i32, "ADataSEG1":i32, "ADataSEG2":i32, "ADataPrescaler":i32, "ADataSJW":i32}}
  T16 = typedef "Blf_Log.ctl" = cluster{"Blf_Log_PATH":path}
  T17 = typedef "UDS Cluster.ctl" = cluster{"UDS Control":T18, "DiagModuleIndex":i32}
  T18 = typedef "UDS Control.ctl" = cluster{"UDS Channel Index":u32, "Request ID":u32, "Response ID":u32, "Request ID (Func)":u32, "Session Mode":u8, "Reset Mode":u8, "DTC Mask":u8, "GropOfDTC":u32, "Seed Level":i32, "Seed":u8[], "Key Level":i32, "Key":u8[], "Read Identifier":u16, "UDS Read Data":u8[], "ASCII Data":string, "Write Identifier":u16, "UDS Wrtie Data":u8[], "IO Control Identifier":u16, "UDS IOControl Data":u8[], "IO Control Mode":u8, "UDS IOControl Read Data":u8[], "Routine Control Identifier":u16, "UDS RoutineControl Data":u8[], "UDS RoutineControl Read Data":u8[], "Routine Control Mode":u8, "SupportFDCAN":bool, "time config":cluster{"p2_timeout":i32, "p2_extended":i32, "s3_servertime":i32, "s3_clienttime":i32}, "ServiceLayer":cluster{"FilledByte":u8, "STMin":i32, "BlockSize":i32, "FCDelay":i32, "MaxLength":i32}, "Request":u8[], "Respond":u8[]}
  T19 = cluster{"Sender":string, "receiver":string, "message":string, "data":variant}
  T20 = typedef "LVPointTypeDef.ctl" = cluster{"Horizontal":i16, "Vertical":i16}
  T21 = cluster{"AChnIndex":u32, "ASupportFDCAN":bool, "AMaxDLC":u16, "ARequestID":u32, "ARequestIDIsStd":bool, "AResponseID":u32, "AResponseIDIsStd":bool, "AFunctionID":u32, "AFunctionIDIsStd":bool}
  T22 = enum32{"invalid app kind", "Development System", "Run Time System", "Student Edition", "Embedded LabVIEW", "Evaluation", "Custom"}
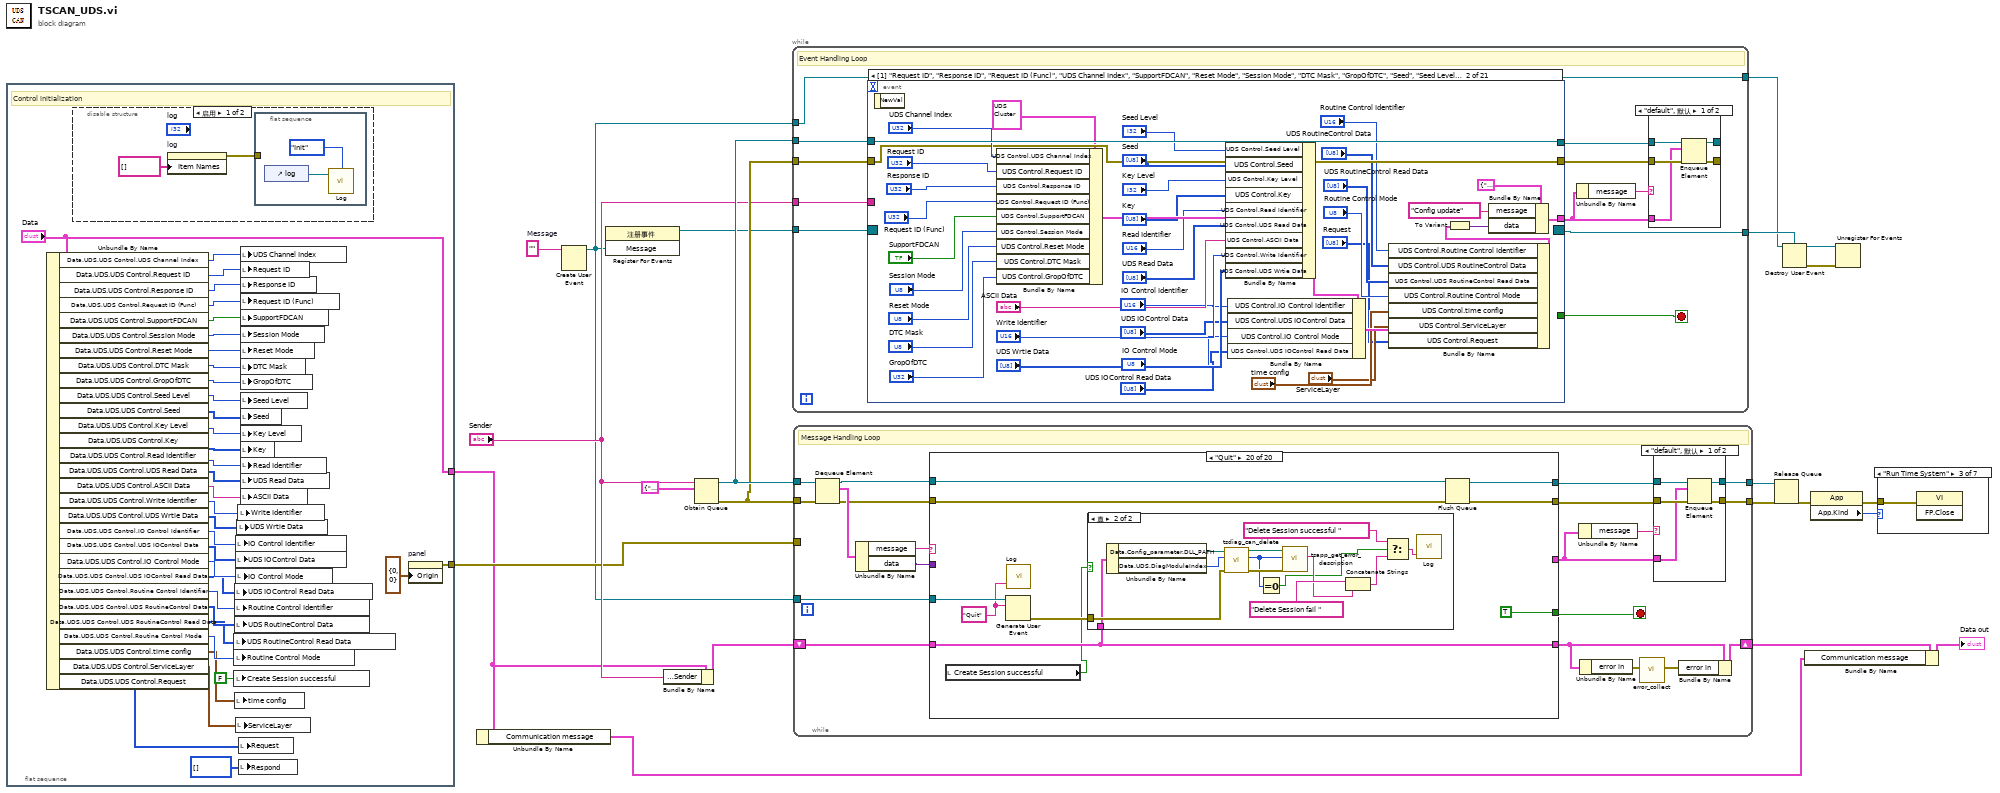
[diagram p0: block diagram]
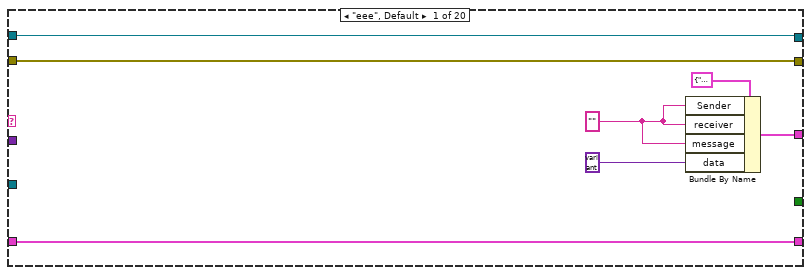
[diagram p10: hidden frame]
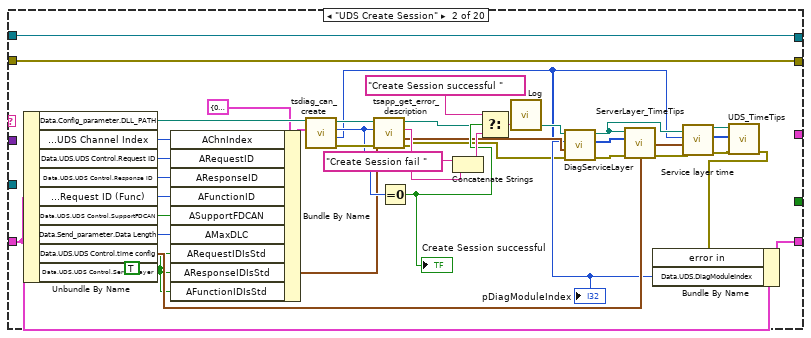
[diagram p11: hidden frame]
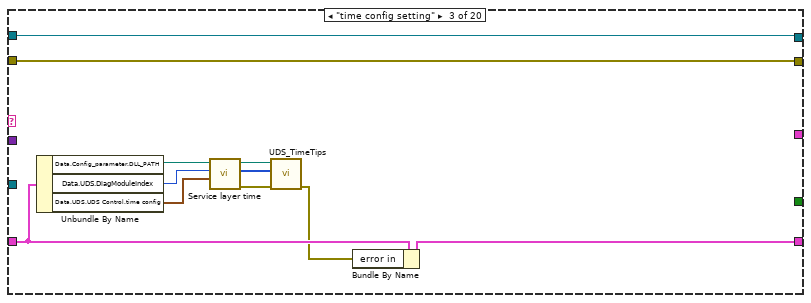
[diagram p12: hidden frame]
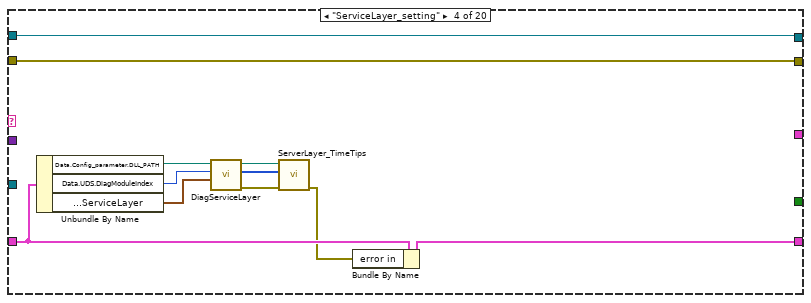
[diagram p13: hidden frame]
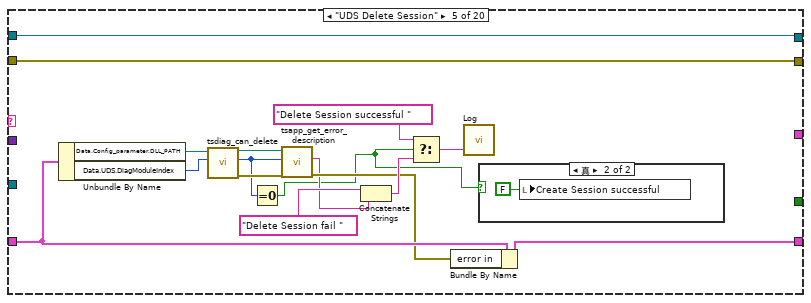
[diagram p14: hidden frame]
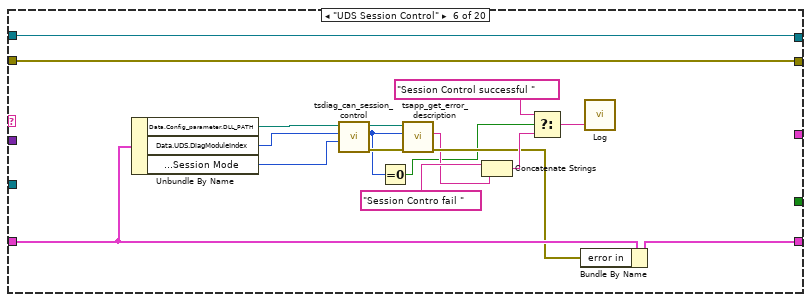
[diagram p16: hidden frame]
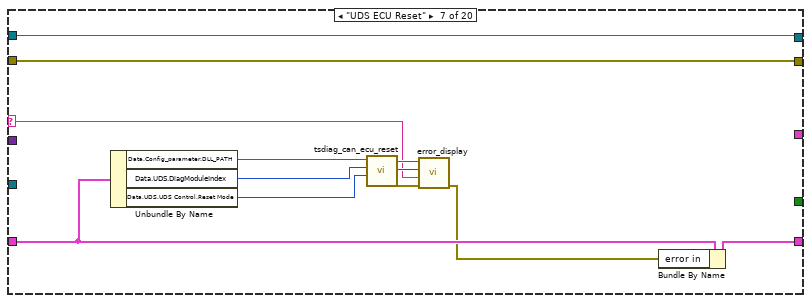
[diagram p17: hidden frame]
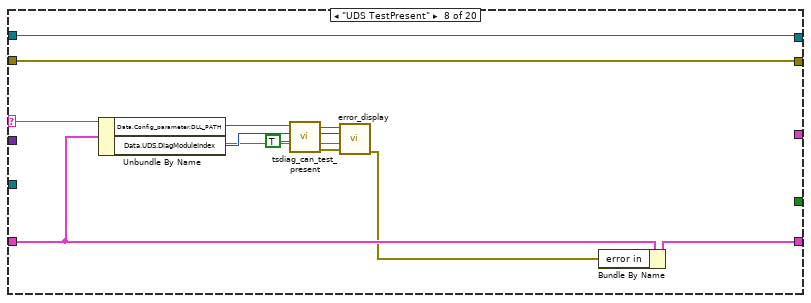
[diagram p18: hidden frame]
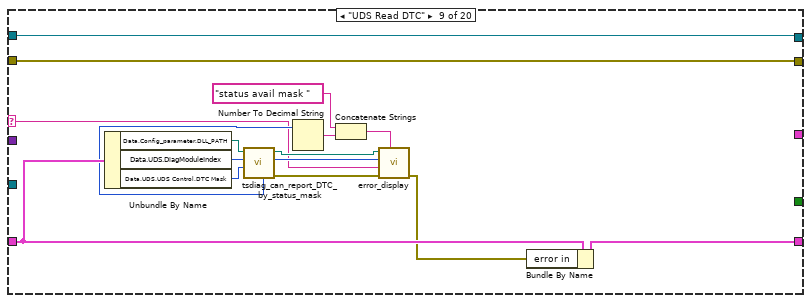
[diagram p19: hidden frame]
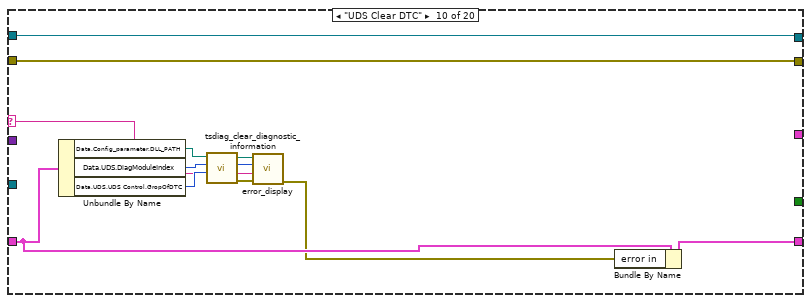
[diagram p20: hidden frame]
diagram:
  w11 = ""  # Message
  n1 = flat-sequence {
    tunnel: [w54] -> w9
    tunnel: ["Data"] -> w2
    frame #0 {
      # "Control initialization"
      n2 = Unbundle By Name("Data") -> ("Data.UDS.UDS Control.UDS Channel Index"=w50:u32, "Data.UDS.UDS Control.Request ID"=w25:u32, "Data.UDS.UDS Control.Response ID"=w26:u32, "Data.UDS.UDS Control.Request ID (Func)"=w52:u32, "Data.UDS.UDS Control.SupportFDCAN"=w51:bool, "Data.UDS.UDS Control.Session Mode"=w49:u8, "Data.UDS.UDS Control.Reset Mode"=w48:u8, "Data.UDS.UDS Control.DTC Mask"=w47:u8, "Data.UDS.UDS Control.GropOfDTC"=w46:u32, "Data.UDS.UDS Control.Seed Level"=w45:i32, "Data.UDS.UDS Control.Seed"=w44:u8[], "Data.UDS.UDS Control.Key Level"=w43:i32, "Data.UDS.UDS Control.Key"=w42:u8[], "Data.UDS.UDS Control.Read Identifier"=w41:u16, "Data.UDS.UDS Control.UDS Read Data"=w40:u8[], "Data.UDS.UDS Control.ASCII Data"=w39:string, "Data.UDS.UDS Control.Write Identifier"=w38:u16, "Data.UDS.UDS Control.UDS Wrtie Data"=w37:u8[], "Data.UDS.UDS Control.IO Control Identifier"=w36:u16, "Data.UDS.UDS Control.UDS IOControl Data"=w35:u8[], "Data.UDS.UDS Control.IO Control Mode"=w34:u8, "Data.UDS.UDS Control.UDS IOControl Read Data"=w33:u8[], "Data.UDS.UDS Control.Routine Control Identifier"=w32:u16, "Data.UDS.UDS Control.UDS RoutineControl Data"=w31:u8[], "Data.UDS.UDS Control.UDS RoutineControl Read Data"=w30:u8[], "Data.UDS.UDS Control.Routine Control Mode"=w29:u8, "Data.UDS.UDS Control.time config"=w27:T2, "Data.UDS.UDS Control.ServiceLayer"=w24:T1, "Data.UDS.UDS Control.Request"=w23:u8[])
      n3 = disable-structure shown="启用" {
        frame Enabled {
          n4 = property on="log" class="LstBox (严格)"("Item Names"=string[] [] ("项名")) -> (error out=w56:errorcluster)  [unwired: 2 in, 1 out]
          n5 = flat-sequence {
            tunnel: w56 -> [_]
            frame #0 {
              n6 = control-ref of="log"() -> (w58:refnum<vi>)
              n7 = call "Log.vi"("Method"=enum16{"Init", "Log"}."Init", "ListBox in"=w58) -> ()  [unwired: 2 in]
            }
          }
        }
        frame Disabled {
        }
      }
      n8 = local write "UDS RoutineControl Read Data"(w30) -> ()
      n9 = local write "Routine Control Mode"(w29) -> ()
      n10 = local write "Create Session successful"(FALSE ("Create Session successful")) -> ()
      n11 = local write "UDS IOControl Read Data"(w33) -> ()
      n12 = local write "Routine Control Identifier"(w32) -> ()
      n13 = local write "UDS RoutineControl Data"(w31) -> ()
      n14 = local write "time config"(w27) -> ()
      n15 = local write "IO Control Identifier"(w36) -> ()
      n16 = local write "UDS IOControl Data"(w35) -> ()
      n17 = local write "IO Control Mode"(w34) -> ()
      n18 = local write "ServiceLayer"(w24) -> ()
      n19 = local write "UDS Wrtie Data"(w37) -> ()
      n20 = local write "Write Identifier"(w38) -> ()
      n21 = local write "Request"(w23) -> ()
      n22 = local write "Respond"(u8[] [] ("Respond")) -> ()
      n23 = local write "UDS Channel Index"(w50) -> ()
      n24 = local write "Request ID"(w25) -> ()
      n25 = local write "Response ID"(w26) -> ()
      n26 = local write "Request ID (Func)"(w52) -> ()
      n27 = local write "SupportFDCAN"(w51) -> ()
      n28 = local write "Session Mode"(w49) -> ()
      n29 = local write "Reset Mode"(w48) -> ()
      n30 = local write "DTC Mask"(w47) -> ()
      n31 = local write "GropOfDTC"(w46) -> ()
      n32 = local write "Seed Level"(w45) -> ()
      n33 = local write "Seed"(w44) -> ()
      n34 = local write "Key Level"(w43) -> ()
      n35 = local write "Key"(w42) -> ()
      n36 = local write "Read Identifier"(w41) -> ()
      n37 = local write "UDS Read Data"(w40) -> ()
      n38 = local write "ASCII Data"(w39) -> ()
      n39 = property on="panel" class="Pane"("Origin"=T20 {"Horizontal"=0, "Vertical"=0} ("原点")) -> (error out=w54:errorcluster)  [unwired: 2 in, 1 out]
    }
  }
  n40 = Unbundle By Name(w2) -> ("Communication message"=w1:T19)
  n41 = Create User Event(user event datatype=w11) -> (user event=w6:refnum<user-event>)  [unwired: 1 in, 1 out]
  n42 = register-events(w6) -> (reference out=w10:refnum<event-registration>)  [unwired: 2 in, 1 out]
  n43 = Bundle By Name(cluster=w2, "Communication message.Sender"="Sender") -> (w13:T3)
  n44 = Obtain Queue(name (unnamed)="Sender", element data type=T19 {"Sender"="", "receiver"="", "message"="", "data"=variant} ("Communication message")) -> (queue out=w21:refnum<queue>, error out=w14:errorcluster)  [unwired: 3 in, 1 out]
  n45 = while {
    tunnel: w21 -> [w69]
    tunnel: w14 -> [w67]
    tunnel: "Sender" -> [w63]
    tunnel: w10 -> [w62]
    tunnel: [w61] -> w8
    tunnel: w6 -> [w60]
    tunnel: [w60] -> w5
    stop <- w70 stop-if-true
    # "Event Handling Loop"
    n46 = event shown="[1] \"Request ID\", \"Response ID\", \"Request ID (Func)\", \"UDS Channel Index\", \"SupportFDCAN\", \"Reset Mode\", \"Session Mode\", \"DTC Mask\", \"GropOfDTC\", \"Seed\", \"Seed Level\", \"Key\", \"Key Level\", \"Read Identifier\", \"UDS Read Data\", \"UDS IOControl Data\", \"UDS IOControl Read Data\", \"Routine Control Identifier\", \"UDS RoutineControl Data\", \"UDS RoutineControl Read Data\", \"Routine Control Mode\", \"IO Control Identifier\", \"IO Control Mode\", \"ASCII Data\", \"Write Identifier\", \"UDS Wrtie Data\", \"time config\", \"ServiceLayer\", \"Request\": 值改变" {
      selector: w62 -> [_ _ _ _ _ _ _ _ _ _ _ _ _ _ _ _ _ _ _ _ _]
      dyn-events: [_ _ _ _ _ _ _ _ _ _ _ _ _ _ _ _ _ _ _ _ _] -> w61
      timeout: _ -> [_ _ _ _ _ _ _ _ _ _ _ _ _ _ _ _ _ _ _ _ _]
      tunnel: [_ _ _ _ _ _ _ _ _ _ _ _ _ _ _ _ _ _ _ w211 w230] -> w70
      tunnel: w69 -> [w80 w120 w125 w130 w135 w140 w145 w150 w155 w160 w165 w170 w175 w180 w185 w190 w195 w200 w207 w214 w232]
      tunnel: [w80 w120 w125 w130 w135 w140 w145 w150 w155 w160 w165 w170 w175 w180 w185 w190 w195 w200 w206 w213 w231] -> w68
      tunnel: [T19 {"Sender"="", "receiver"="", "message"="", "data"=variant} ("Communication message") w117 w122 w126 w131 w137 w142 w146 w151 w156 w161 w166 w171 w176 w181 w186 w191 w196 w209 _ _] -> w65
      tunnel: [w79 w111 w121 w129 w134 w136 w141 w149 w154 w159 w164 w169 w174 w179 w184 w189 w194 w199 w204 w212 w228] -> w66
      tunnel: w67 -> [w79 w111 w121 w129 w134 w136 w141 w149 w154 w159 w164 w169 w174 w179 w184 w189 w194 w199 w205 w215 w229]
      tunnel: w63 -> [_ _ _ _ _ _ _ _ _ _ _ _ _ _ _ _ _ _ _ _ _]
      event Timeout {
        n47 = event-data() -> ()  [unwired: 1 in, 3 out]
      }
      event "Request ID", "Response ID", "Request ID (Func)", "UDS Channel Index", "SupportFDCAN", "Reset Mode", "Session Mode", "DTC Mask", "GropOfDTC", "Seed", "Seed Level", "Key", "Key Level", "Read Identifier", "UDS Read Data", "UDS IOControl Data", "UDS IOControl Read Data", "Routine Control Identifier", "UDS RoutineControl Data", "UDS RoutineControl Read Data", "Routine Control Mode", "IO Control Identifier", "IO Control Mode", "ASCII Data", "Write Identifier", "UDS Wrtie Data", "time config", "ServiceLayer", "Request": Value Change {
        n48 = event-data() -> ()  [unwired: 1 in, 1 out]
        n49 = Bundle By Name(cluster=T17 {"UDS Control"={"UDS Channel Index"=0, "Request ID"=1984, "Response ID"=1992, "Request ID (Func)"=2015, "Session Mode"=1, "Reset Mode"=1, "DTC Mask"=255, "GropOfDTC"=16777215, "Seed Level"=1, "Seed"=[], "Key Level"=2, "Key"=[], "Read Identifier"=0, "UDS Read Data"=[], "ASCII Data"="", "Write Identifier"=0, "UDS Wrtie Data"=[], "IO Control Identifier"=0, "UDS IOControl Data"=[], "IO Control Mode"=0, "UDS IOControl Read Data"=[], "Routine Control Identifier"=0, "UDS RoutineControl Data"=[], "UDS RoutineControl Read Data"=[], "Routine Control Mode"=1, "SupportFDCAN"=TRUE, "time config"={"p2_timeout"=0, "p2_extended"=0, "s3_servertime"=0, "s3_clienttime"=0}, "ServiceLayer"={"FilledByte"=0, "STMin"=10, "BlockSize"=10, "FCDelay"=10, "MaxLength"=4095}, "Request"=[], "Respond"=[]}, "DiagModuleIndex"=0} ("UDS"), "UDS Control.UDS Channel Index"="UDS Channel Index", "UDS Control.Request ID"="Request ID", "UDS Control.Response ID"="Response ID", "UDS Control.Request ID (Func)"="Request ID (Func)", "UDS Control.SupportFDCAN"="SupportFDCAN", "UDS Control.Session Mode"="Session Mode", "UDS Control.Reset Mode"="Reset Mode", "UDS Control.DTC Mask"="DTC Mask", "UDS Control.GropOfDTC"="GropOfDTC") -> (w113:T17)
        n50 = Bundle By Name(cluster=w113, "UDS Control.Seed Level"="Seed Level", "UDS Control.Seed"="Seed", "UDS Control.Key Level"="Key Level", "UDS Control.Key"="Key", "UDS Control.Read Identifier"="Read Identifier", "UDS Control.UDS Read Data"="UDS Read Data", "UDS Control.ASCII Data"="ASCII Data", "UDS Control.Write Identifier"="Write Identifier", "UDS Control.UDS Wrtie Data"="UDS Wrtie Data") -> (w98:T17)
        n51 = Bundle By Name(cluster=w98, "UDS Control.IO Control Identifier"="IO Control Identifier", "UDS Control.UDS IOControl Data"="UDS IOControl Data", "UDS Control.IO Control Mode"="IO Control Mode", "UDS Control.UDS IOControl Read Data"="UDS IOControl Read Data") -> (w93:T17)
        n52 = Bundle By Name(cluster=w93, "UDS Control.Routine Control Identifier"="Routine Control Identifier", "UDS Control.UDS RoutineControl Data"="UDS RoutineControl Data", "UDS Control.UDS RoutineControl Read Data"="UDS RoutineControl Read Data", "UDS Control.Routine Control Mode"="Routine Control Mode", "UDS Control.time config"="time config", "UDS Control.ServiceLayer"="ServiceLayer", "UDS Control.Request"="Request") -> (w92:T17)
        n53 = To Variant(anything=w92) -> (Variant=w114:variant)
        n54 = Bundle By Name(cluster=T19 {"Sender"="", "receiver"="", "message"="", "data"=variant} ("Communication message"), "message"="Config update" ("Sender"), "data"=w114) -> (w117:T19)
      }
      event "UDS Create Session": Value Change {
        n55 = event-data() -> ()  [unwired: 1 in, 6 out]
        n56 = Bundle By Name(cluster=T19 {"Sender"="", "receiver"="", "message"="", "data"=variant} ("Communication message"), "message"="UDS Create Session" ("Sender")) -> (w122:T19)
      }
      event "time config setting": Value Change {
        n57 = event-data() -> ()  [unwired: 1 in, 6 out]
        n58 = Bundle By Name(cluster=T19 {"Sender"="", "receiver"="", "message"="", "data"=variant} ("Communication message"), "message"="time config setting" ("Sender")) -> (w126:T19)
      }
      event "ServiceLayer_setting": Value Change {
        n59 = event-data() -> ()  [unwired: 1 in, 6 out]
        n60 = Bundle By Name(cluster=T19 {"Sender"="", "receiver"="", "message"="", "data"=variant} ("Communication message"), "message"="ServiceLayer_setting" ("Sender")) -> (w131:T19)
      }
      event "UDS Delete Session": Value Change {
        n61 = event-data() -> ()  [unwired: 1 in, 6 out]
        n62 = Bundle By Name(cluster=T19 {"Sender"="", "receiver"="", "message"="", "data"=variant} ("Communication message"), "message"="UDS Delete Session" ("Sender")) -> (w137:T19)
      }
      event "UDS Session Control": Value Change {
        n63 = event-data() -> ()  [unwired: 1 in, 6 out]
        n64 = Bundle By Name(cluster=T19 {"Sender"="", "receiver"="", "message"="", "data"=variant} ("Communication message"), "message"="UDS Session Control" ("Sender")) -> (w142:T19)
      }
      event "UDS ECU Reset": Value Change {
        n65 = event-data() -> ()  [unwired: 1 in, 6 out]
        n66 = Bundle By Name(cluster=T19 {"Sender"="", "receiver"="", "message"="", "data"=variant} ("Communication message"), "message"="UDS ECU Reset" ("Sender")) -> (w146:T19)
      }
      event "UDS TestPresent": Value Change {
        n67 = event-data() -> ()  [unwired: 1 in, 6 out]
        n68 = Bundle By Name(cluster=T19 {"Sender"="", "receiver"="", "message"="", "data"=variant} ("Communication message"), "message"="UDS TestPresent" ("Sender")) -> (w151:T19)
      }
      event "UDS Read DTC": Value Change {
        n69 = event-data() -> ()  [unwired: 1 in, 6 out]
        n70 = Bundle By Name(cluster=T19 {"Sender"="", "receiver"="", "message"="", "data"=variant} ("Communication message"), "message"="UDS Read DTC" ("Sender")) -> (w156:T19)
      }
      event "UDS Clear DTC": Value Change {
        n71 = event-data() -> ()  [unwired: 1 in, 6 out]
        n72 = Bundle By Name(cluster=T19 {"Sender"="", "receiver"="", "message"="", "data"=variant} ("Communication message"), "message"="UDS Clear DTC" ("Sender")) -> (w161:T19)
      }
      event "UDS Request Seed": Value Change {
        n73 = event-data() -> ()  [unwired: 1 in, 6 out]
        n74 = Bundle By Name(cluster=T19 {"Sender"="", "receiver"="", "message"="", "data"=variant} ("Communication message"), "message"="UDS Request Seed" ("Sender")) -> (w166:T19)
      }
      event "UDS Send Key": Value Change {
        n75 = event-data() -> ()  [unwired: 1 in, 6 out]
        n76 = Bundle By Name(cluster=T19 {"Sender"="", "receiver"="", "message"="", "data"=variant} ("Communication message"), "message"="UDS Send Key" ("Sender")) -> (w171:T19)
      }
      event "UDS Read by Identifier": Value Change {
        n77 = event-data() -> ()  [unwired: 1 in, 6 out]
        n78 = Bundle By Name(cluster=T19 {"Sender"="", "receiver"="", "message"="", "data"=variant} ("Communication message"), "message"="UDS Read by Identifier" ("Sender")) -> (w176:T19)
      }
      event "UDS Write by Identifier": Value Change {
        n79 = event-data() -> ()  [unwired: 1 in, 6 out]
        n80 = Bundle By Name(cluster=T19 {"Sender"="", "receiver"="", "message"="", "data"=variant} ("Communication message"), "message"="UDS Write by Identifier" ("Sender")) -> (w181:T19)
      }
      event "UDS IOControl by Identifier": Value Change {
        n81 = event-data() -> ()  [unwired: 1 in, 6 out]
        n82 = Bundle By Name(cluster=T19 {"Sender"="", "receiver"="", "message"="", "data"=variant} ("Communication message"), "message"="UDS IOControl by Identifier" ("Sender")) -> (w186:T19)
      }
      event "UDS RoutineControl by Identifier": Value Change {
        n83 = event-data() -> ()  [unwired: 1 in, 6 out]
        n84 = Bundle By Name(cluster=T19 {"Sender"="", "receiver"="", "message"="", "data"=variant} ("Communication message"), "message"="UDS RoutineControl by Identifier" ("Sender")) -> (w191:T19)
      }
      event "UDS Execute": Value Change {
        n85 = event-data() -> ()  [unwired: 1 in, 6 out]
        n86 = Bundle By Name(cluster=T19 {"Sender"="", "receiver"="", "message"="", "data"=variant} ("Communication message"), "message"="UDS Execute" ("Sender")) -> (w196:T19)
      }
      event "Quit": Value Change {
        n87 = event-data() -> ()  [unwired: 1 in, 6 out]
        n88 = Bundle By Name(cluster=T19 {"Sender"="", "receiver"="", "message"="", "data"=variant} ("Communication message"), "message"="UDS Delete Session" ("Sender")) -> (w201:T19)
        n89 = Enqueue Element(queue=w207, element=w201, error in (no error)=w205) -> (queue out=w206:refnum<queue>, error out=w204:errorcluster)  [unwired: 1 in, 1 out]
        n90 = Bundle By Name(cluster=T19 {"Sender"="", "receiver"="", "message"="", "data"=variant} ("Communication message"), "message"="Quit" ("Sender")) -> (w209:T19)
      }
      event User Event {
        n91 = event-data() -> ("Message"=w217:string)  [unwired: 1 in]
        n92 = Equal?(x=w217, y="Quit") -> (x = y?=w211:bool)
        n93 = case shown="真" w211 {
          tunnel: w215 -> [w218 w223]
          tunnel: w214 -> [w219 w222]
          tunnel: [w219 w221] -> w213
          tunnel: [w218 w220] -> w212
          frame False {
          }
          frame True {
            n94 = Bundle By Name(cluster=T19 {"Sender"="", "receiver"="", "message"="", "data"=variant} ("Communication message"), "message"="UDS Delete Session" ("Sender")) -> (w224:T19)
            n95 = Enqueue Element(queue=w222, element=w224, error in (no error)=w223) -> (queue out=w221:refnum<queue>, error out=w220:errorcluster)  [unwired: 1 in, 1 out]
          }
        }
      }
      event Panel Close? {
        w230 = TRUE ("放弃？")
        n96 = event-data() -> ()  [unwired: 1 in, 4 out]
        n97 = for {
          shift-right: [w238] -> w231
          shift-left: w232 -> [w239]
          shift-right: [w234] -> w228
          shift-left: w229 -> [w235]
          tunnel: string[] ["UDS Delete Session", "Quit"] -> [w233] mode=indexing
          n98 = Bundle By Name(cluster=T19 {"Sender"="", "receiver"="", "message"="", "data"=variant} ("Communication message"), "message"=w233) -> (w236:T19)
          n99 = Enqueue Element(queue=w239, element=w236, error in (no error)=w235) -> (queue out=w238:refnum<queue>, error out=w234:errorcluster)  [unwired: 1 in, 1 out]
        }
        n100 = event-data("Discard?"=w230) -> ()  [unwired: 1 in, 1 out]
      }
    }
    n101 = Unbundle By Name(w65) -> ("message"=w64:string)
    n102 = case shown="\"default\", 默认" w64 {
      tunnel: w68 -> [w75 w77]
      tunnel: w66 -> [w74 w76]
      tunnel: w65 -> [w73 _]
      tunnel: [w72 w77] -> _
      tunnel: [w71 w76] -> _
      frame "default", Default {
        n103 = Enqueue Element(queue=w75, element=w73, error in (no error)=w74) -> (queue out=w72:refnum<queue>, error out=w71:errorcluster)  [unwired: 1 in, 1 out]
      }
      frame "" {
      }
    }
  }
  n104 = while {
    tunnel: w21 -> [w259]
    tunnel: w14 -> [w258]
    tunnel: [w250] -> w20
    tunnel: [w249] -> w19
    shift-right: [w241] -> w4
    shift-left: w13 -> [w245]
    tunnel: w9 -> [_]
    tunnel: w6 -> [w244]
    stop <- w248 stop-if-true
    # "Message Handling Loop"
    n105 = Dequeue Element(queue=w259, error in (no error)=w258) -> (queue out=w255:refnum<queue>, element=w257:T19, error out=w254:errorcluster)  [unwired: 1 in, 1 out]
    n106 = Unbundle By Name(w257) -> ("message"=w256:string, "data"=w251:variant)
    n107 = case shown="\"Quit\"" w256 {
      selector: w256 -> [_ _ _ _ _ _ w368 w380 w390 w406 w419 w440 w452 w474 w487 _ w542 _ _ _]
      tunnel: [w273 w294 w320 w331 w337 w354 w377 w389 w405 w417 w431 w451 w465 w486 w502 w530 w551 w556 w562 w571] -> w253
      tunnel: w255 -> [w273 w294 w320 w331 w337 w354 w377 w389 w405 w417 w431 w451 w465 w486 w502 w530 w551 w556 w562 w570]
      tunnel: w254 -> [w272 w293 w319 w330 w336 w353 w376 w388 w404 w416 w430 w450 w464 w485 w501 w529 w550 w555 w561 w568]
      tunnel: [w272 w293 w319 w330 w336 w353 w376 w388 w404 w416 w430 w450 w464 w485 w501 w529 w550 w555 w561 w569] -> w252
      tunnel: w251 -> [_ _ _ _ _ _ _ _ _ _ _ _ _ _ _ _ _ w559 _ _]
      tunnel: [_ _ _ _ _ _ _ _ _ _ _ _ _ _ _ _ _ _ _ TRUE] -> w248
      tunnel: [w270 _ _ _ _ _ _ _ _ _ _ _ _ _ _ _ _ _ _ _] -> w247
      tunnel: [w267 w300 w314 w328 w339 w356 w371 w383 w399 w411 w425 w444 w459 w480 w494 w522 w541 w557 w560 w564] -> w243
      tunnel: w245 -> [w267 w309 w318 w329 w347 w365 w375 w387 w403 w415 w429 w449 w463 w484 w500 w528 w549 w558 w560 w564]
      tunnel: w244 -> [_ _ _ _ _ _ _ _ _ _ _ _ _ _ _ _ _ _ _ w567]
      frame "eee", Default {
        w268 = ""
        n108 = Bundle By Name(cluster=T19 {"Sender"="", "receiver"="", "message"="", "data"=variant} ("Communication message"), "Sender"=w268, "receiver"=w268, "message"=w268, "data"=variant) -> (w270:T19)
      }
      frame "UDS Create Session" {
        w287 = TRUE ("ARequestIDIsStd")
        n109 = Unbundle By Name(w309) -> ("Data.Config_parameter.DLL_PATH"=w308:path, "Data.UDS.UDS Control.UDS Channel Index"=w305:u32, "Data.UDS.UDS Control.Request ID"=w303:u32, "Data.UDS.UDS Control.Response ID"=w302:u32, "Data.UDS.UDS Control.Request ID (Func)"=w301:u32, "Data.UDS.UDS Control.SupportFDCAN"=w304:bool, "Data.Send_parameter.Data Length"=w286:i32, "Data.UDS.UDS Control.time config"=w290:T2, "Data.UDS.UDS Control.ServiceLayer"=w280:T1)
        n110 = Bundle By Name(cluster=T21 {"AChnIndex"=0, "ASupportFDCAN"=FALSE, "AMaxDLC"=0, "ARequestID"=0, "ARequestIDIsStd"=FALSE, "AResponseID"=0, "AResponseIDIsStd"=FALSE, "AFunctionID"=0, "AFunctionIDIsStd"=FALSE} ("Cluster"), "AChnIndex"=w305, "ARequestID"=w303, "AResponseID"=w302, "AFunctionID"=w301, "ASupportFDCAN"=w304, "AMaxDLC"=w286, "ARequestIDIsStd"=w287, "AResponseIDIsStd"=w287, "AFunctionIDIsStd"=w287) -> (w306:T21)
        n111 = call "tsdiag_can_create.vi"("Cluster"=w306, "path"=w308) -> ("错误输出"=w299:errorcluster, "pDiagModuleIndex"=w275:i32, "Return Type"=w289:i32, "path output"=w292:path)  [unwired: 6 in]
        "pDiagModuleIndex" <- w275
        n112 = call "tsapp_get_error_description.vi"("error in"=w299, "ACount"=w289, "路径输入"=w292) -> ("error out"=w274:errorcluster, "ErrDes"=w291:string, "路径输出"=w281:path)  [unwired: 6 in]
        n113 = Equal To 0?(x=w289) -> (x = 0?=w288:bool)
        "Create Session successful" <- w288
        n114 = Concatenate Strings("Create Session fail ", w291) -> (w297:string)
        n115 = Select(t="Create Session successful ", s=w288, f=w297) -> (s? t:f=w295:string)
        n116 = call "Log.vi"("Data"=w295) -> ()  [unwired: 3 in]
        n117 = call "DiagServiceLayer.vi"("path"=w281, "ADiagModuleIndex"=w275, "Diag传输层参数"=w280, "错误输入"=w274) -> ("path out"=w279:path, "returns"=w277:i32[], "错误输出"=w276:errorcluster)  [unwired: 4 in]
        n118 = call "ServerLayer_TimeTips.vi"("error in"=w276, "result array"=w277, "path"=w279) -> ("错误输出"=w278:errorcluster)  [unwired: 7 in, 1 out]
        n119 = call "Service layer time.vi"("error in (no error)"=w278, "time config"=w290, "ADiagModuleIndex"=w275, "路径输入"=w279) -> ("error out"=w284:errorcluster, "returns"=w283:i32[], "路径输出"=w285:path)  [unwired: 5 in]
        n120 = call "UDS_TimeTips.vi"("error in"=w284, "result array"=w283, "path"=w285) -> ("错误输出"=w282:errorcluster)  [unwired: 7 in, 1 out]
        n121 = Bundle By Name(cluster=w309, "error in"=w282, "Data.UDS.DiagModuleIndex"=w275) -> (w300:T3)
      }
      frame "time config setting" {
        n122 = Unbundle By Name(w318) -> ("Data.Config_parameter.DLL_PATH"=w317:path, "Data.UDS.DiagModuleIndex"=w316:i32, "Data.UDS.UDS Control.time config"=w315:T2)
        n123 = call "Service layer time.vi"("time config"=w315, "ADiagModuleIndex"=w316, "路径输入"=w317) -> ("error out"=w311:errorcluster, "returns"=w312:i32[], "路径输出"=w313:path)  [unwired: 6 in]
        n124 = call "UDS_TimeTips.vi"("error in"=w311, "result array"=w312, "path"=w313) -> ("错误输出"=w310:errorcluster)  [unwired: 7 in, 1 out]
        n125 = Bundle By Name(cluster=w318, "error in"=w310) -> (w314:T3)
      }
      frame "ServiceLayer_setting" {
        n126 = Unbundle By Name(w329) -> ("Data.Config_parameter.DLL_PATH"=w327:path, "Data.UDS.DiagModuleIndex"=w326:i32, "Data.UDS.UDS Control.ServiceLayer"=w325:T1)
        n127 = call "DiagServiceLayer.vi"("path"=w327, "ADiagModuleIndex"=w326, "Diag传输层参数"=w325) -> ("path out"=w324:path, "returns"=w323:i32[], "错误输出"=w322:errorcluster)  [unwired: 5 in]
        n128 = call "ServerLayer_TimeTips.vi"("error in"=w322, "result array"=w323, "path"=w324) -> ("错误输出"=w321:errorcluster)  [unwired: 7 in, 1 out]
        n129 = Bundle By Name(cluster=w329, "error in"=w321) -> (w328:T3)
      }
      frame "UDS Delete Session" {
        n130 = Unbundle By Name(w347) -> ("Data.Config_parameter.DLL_PATH"=w346:path, "Data.UDS.DiagModuleIndex"=w345:i32)
        n131 = call "tsdiag_can_delete.vi"("ADiagModuleIndex"=w345, "path"=w346) -> ("错误输出"=w340:errorcluster, "Return Type"=w333:i32, "path out"=w335:path)  [unwired: 7 in]
        n132 = Equal To 0?(x=w333) -> (x = 0?=w332:bool)
        n133 = call "tsapp_get_error_description.vi"("error in"=w340, "ACount"=w333, "路径输入"=w335) -> ("error out"=w338:errorcluster, "ErrDes"=w334:string)  [unwired: 6 in, 1 out]
        n134 = Concatenate Strings("Delete Session fail ", w334) -> (w343:string)
        n135 = Select(t="Delete Session successful ", s=w332, f=w343) -> (s? t:f=w341:string)
        n136 = Bundle By Name(cluster=w347, "error in"=w338) -> (w339:T3)
        n137 = call "Log.vi"("Data"=w341) -> ()  [unwired: 3 in]
        n138 = case shown="真" w332 {
          frame False {
          }
          frame True {
            n139 = local write "Create Session successful"(FALSE ("Create Session successful")) -> ()
          }
        }
      }
      frame "UDS Session Control" {
        n140 = Unbundle By Name(w365) -> ("Data.Config_parameter.DLL_PATH"=w364:path, "Data.UDS.DiagModuleIndex"=w363:i32, "Data.UDS.UDS Control.Session Mode"=w362:u8)
        n141 = call "tsdiag_can_session_control.vi"("ASubSession"=w362, "ADiagModuleIndex"=w363, "path"=w364) -> ("错误输出"=w357:errorcluster, "Return Type"=w350:i32, "path out"=w352:path)  [unwired: 6 in]
        n142 = Equal To 0?(x=w350) -> (x = 0?=w349:bool)
        n143 = call "tsapp_get_error_description.vi"("error in"=w357, "ACount"=w350, "路径输入"=w352) -> ("error out"=w355:errorcluster, "ErrDes"=w351:string)  [unwired: 6 in, 1 out]
        n144 = Concatenate Strings("Session Contro fail ", w351) -> (w360:string)
        n145 = Select(t="Session Control successful ", s=w349, f=w360) -> (s? t:f=w358:string)
        n146 = Bundle By Name(cluster=w365, "error in"=w355) -> (w356:T3)
        n147 = call "Log.vi"("Data"=w358) -> ()  [unwired: 3 in]
      }
      frame "UDS ECU Reset" {
        n148 = Unbundle By Name(w375) -> ("Data.Config_parameter.DLL_PATH"=w374:path, "Data.UDS.DiagModuleIndex"=w373:i32, "Data.UDS.UDS Control.Reset Mode"=w372:u8)
        n149 = call "tsdiag_can_ecu_reset.vi"("mode"=w372, "ADiagModuleIndex"=w373, "path"=w374) -> ("error out"=w367:errorcluster, "Return Type"=w369:i32, "path out"=w370:path)  [unwired: 4 in, 2 out]
        n150 = call "error_display.vi"("error in"=w367, "Action name"=w368, "return"=w369, "DLL path"=w370) -> ("error out"=w366:errorcluster)  [unwired: 6 in, 1 out]
        n151 = Bundle By Name(cluster=w375, "error in"=w366) -> (w371:T3)
      }
      frame "UDS TestPresent" {
        n152 = Unbundle By Name(w387) -> ("Data.Config_parameter.DLL_PATH"=w386:path, "Data.UDS.DiagModuleIndex"=w385:i32)
        n153 = call "tsdiag_can_test_present.vi"("response required?"=TRUE, "ADiagModuleIndex"=w385, "路径输入"=w386) -> ("error out"=w379:errorcluster, "Return Type"=w381:i32, "路径输出"=w382:path)  [unwired: 5 in, 1 out]
        n154 = call "error_display.vi"("error in"=w379, "Action name"=w380, "return"=w381, "DLL path"=w382) -> ("error out"=w378:errorcluster)  [unwired: 6 in, 1 out]
        n155 = Bundle By Name(cluster=w387, "error in"=w378) -> (w383:T3)
      }
      frame "UDS Read DTC" {
        n156 = Unbundle By Name(w403) -> ("Data.Config_parameter.DLL_PATH"=w402:path, "Data.UDS.DiagModuleIndex"=w401:i32, "Data.UDS.UDS Control.DTC Mask"=w400:u8)
        n157 = call "tsdiag_can_report_DTC_by_status_mask.vi"("status mask"=w400, "ADiagModuleIndex"=w401, "path"=w402) -> ("error out"=w393:errorcluster, "Return Type"=w394:i32, "path out"=w395:path, "status avail mask"=w397:u8)  [unwired: 3 in, 2 out]
        n158 = Number To Decimal String(number=w397) -> (decimal integer string=w396:string)  [unwired: 1 in]
        n159 = Concatenate Strings("status avail mask ", w396) -> (w391:string)
        n160 = call "error_display.vi"("OK_add"=w391, "error in"=w393, "Action name"=w390, "return"=w394, "DLL path"=w395) -> ("error out"=w392:errorcluster)  [unwired: 5 in, 1 out]
        n161 = Bundle By Name(cluster=w403, "error in"=w392) -> (w399:T3)
      }
      frame "UDS Clear DTC" {
        n162 = Unbundle By Name(w415) -> ("Data.Config_parameter.DLL_PATH"=w414:path, "Data.UDS.DiagModuleIndex"=w413:i32, "Data.UDS.UDS Control.GropOfDTC"=w412:u32)
        n163 = call "tsdiag_clear_diagnostic_information.vi"("group of DTC"=w412, "ADiagModuleIndex"=w413, "path"=w414) -> ("error out"=w408:errorcluster, "Return Type"=w409:i32, "path out"=w410:path)  [unwired: 5 in, 1 out]
        n164 = call "error_display.vi"("error in"=w408, "Action name"=w406, "return"=w409, "DLL path"=w410) -> ("error out"=w407:errorcluster)  [unwired: 6 in, 1 out]
        n165 = Bundle By Name(cluster=w415, "error in"=w407) -> (w411:T3)
      }
      frame "UDS Request Seed" {
        n166 = Unbundle By Name(w429) -> ("Data.Config_parameter.DLL_PATH"=w428:path, "Data.UDS.DiagModuleIndex"=w427:i32, "Data.UDS.UDS Control.Seed Level"=w426:i32)
        n167 = call "tsdiag_can_security_access_request_seed.vi"("ALevel"=w426, "ADiagModuleIndex"=w427, "path"=w428) -> ("错误输出"=w421:errorcluster, "ARecSeed"=w424:u8[], "Return Type"=w420:i32, "path out"=w422:path)  [unwired: 5 in]
        n168 = call "error_display.vi"("error in"=w421, "Action name"=w419, "return"=w420, "DLL path"=w422) -> ("error out"=w418:errorcluster)  [unwired: 6 in, 1 out]
        n169 = Equal To 0?(x=w420) -> (x = 0?=w423:bool)
        n170 = case shown="假" w423 {
          tunnel: w429 -> [w434 w438]
          tunnel: [w433 w437] -> w425
          tunnel: w424 -> [_ w436]
          tunnel: w418 -> [w432 w435]
          frame False {
            n171 = Bundle By Name(cluster=w434, "error in"=w432) -> (w433:T3)
          }
          frame True {
            n172 = local write "Seed"(w436) -> ()
            n173 = Bundle By Name(cluster=w438, "error in"=w435, "Data.UDS.UDS Control.Seed"=w436) -> (w437:T3)
          }
        }
      }
      frame "UDS Send Key" {
        n174 = Unbundle By Name(w449) -> ("Data.Config_parameter.DLL_PATH"=w448:path, "Data.UDS.DiagModuleIndex"=w447:i32, "Data.UDS.UDS Control.Key Level"=w446:i32, "Data.UDS.UDS Control.Key"=w445:u8[])
        n175 = call "tsdiag_can_security_access_send_key.vi"("AKeyValue"=w445, "ALevel"=w446, "ADiagModuleIndex"=w447, "path"=w448) -> ("错误输出"=w442:errorcluster, "Return Type"=w441:i32, "path out"=w443:path)  [unwired: 5 in]
        n176 = call "error_display.vi"("error in"=w442, "Action name"=w440, "return"=w441, "DLL path"=w443) -> ("error out"=w439:errorcluster)  [unwired: 6 in, 1 out]
        n177 = Bundle By Name(cluster=w449, "error in"=w439) -> (w444:T3)
      }
      frame "UDS Read by Identifier" {
        # "Read diagnostic information based on ID"
        n178 = Unbundle By Name(w463) -> ("Data.Config_parameter.DLL_PATH"=w462:path, "Data.UDS.DiagModuleIndex"=w461:i32, "Data.UDS.UDS Control.Read Identifier"=w460:u16)
        n179 = call "tsdiag_can_read_data_by_identifier.vi"("ADataIdentifier"=w460, "ADiagModuleIndex"=w461, "路径输入"=w462) -> ("error out"=w454:errorcluster, "Data"=w458:u8[], "return"=w455:i32, "路径输出"=w456:path)  [unwired: 5 in]
        n180 = Equal To 0?(x=w455) -> (x = 0?=w457:bool)
        n181 = call "error_display.vi"("error in"=w454, "Action name"=w452, "return"=w455, "DLL path"=w456) -> ("error out"=w453:errorcluster)  [unwired: 6 in, 1 out]
        n182 = case shown="假" w457 {
          tunnel: w463 -> [w468 w473]
          tunnel: [w467 w472] -> w459
          tunnel: w458 -> [_ w471]
          tunnel: w453 -> [w466 w469]
          frame False {
            n183 = Bundle By Name(cluster=w468, "error in"=w466) -> (w467:T3)
          }
          frame True {
            n184 = Byte Array To String(unsigned byte array=w471) -> (string=w470:string)
            n185 = local write "ASCII Data"(w470) -> ()
            n186 = local write "UDS Read Data"(w471) -> ()
            n187 = Bundle By Name(cluster=w473, "error in"=w469, "Data.UDS.UDS Control.UDS Read Data"=w471, "Data.UDS.UDS Control.ASCII Data"=w470) -> (w472:T3)
          }
        }
      }
      frame "UDS Write by Identifier" {
        # "Write diagnostic information based on ID"
        n188 = Unbundle By Name(w484) -> ("Data.Config_parameter.DLL_PATH"=w483:path, "Data.UDS.DiagModuleIndex"=w482:i32, "Data.UDS.UDS Control.Write Identifier"=w481:u16, "Data.UDS.UDS Control.UDS Wrtie Data"=w479:u8[])
        n189 = call "tsdiag_can_write_data_by_identifier.vi"("Data"=w479, "ADataIdentifier"=w481, "ADiagModuleIndex"=w482, "路径输入"=w483) -> ("error out"=w476:errorcluster, "return"=w477:i32, "路径输出"=w478:path)  [unwired: 5 in]
        n190 = call "error_display.vi"("error in"=w476, "Action name"=w474, "return"=w477, "DLL path"=w478) -> ("error out"=w475:errorcluster)  [unwired: 6 in, 1 out]
        n191 = Bundle By Name(cluster=w484, "error in"=w475) -> (w480:T3)
      }
      frame "UDS IOControl by Identifier" {
        n192 = Unbundle By Name(w500) -> ("Data.UDS.UDS Control.IO Control Mode"=w495:u8, "Data.Config_parameter.DLL_PATH"=w499:path, "Data.UDS.DiagModuleIndex"=w498:i32, "Data.UDS.UDS Control.IO Control Identifier"=w497:u16, "Data.UDS.UDS Control.UDS IOControl Data"=w496:u8[])
        n193 = call "tsdiag_can_input_output_control_by_identifier.vi"("data in"=w496, "mode"=w495, "ID"=w497, "ADiagModuleIndex"=w498, "path"=w499) -> ("error out"=w489:errorcluster, "success?"=w492:bool, "Return Type"=w490:i32, "path out"=w491:path, "data out"=w493:u8[])  [unwired: 2 in]
        n194 = call "error_display.vi"("error in"=w489, "Action name"=w487, "return"=w490, "DLL path"=w491) -> ("error out"=w488:errorcluster)  [unwired: 6 in, 1 out]
        n195 = case shown="真" w492 {
          tunnel: w500 -> [w505 w509]
          tunnel: [w504 w508] -> w494
          tunnel: w493 -> [_ w507]
          tunnel: w488 -> [w503 w506]
          frame False {
            n196 = Bundle By Name(cluster=w505, "error in"=w503) -> (w504:T3)
          }
          frame True {
            n197 = local write "UDS IOControl Read Data"(w507) -> ()
            n198 = Bundle By Name(cluster=w509, "error in"=w506, "Data.UDS.UDS Control.UDS IOControl Read Data"=w507) -> (w508:T3)
          }
        }
      }
      frame "UDS RoutineControl by Identifier" {
        n199 = Unbundle By Name(w528) -> ("Data.UDS.UDS Control.Routine Control Mode"=w526:u8, "Data.Config_parameter.DLL_PATH"=w527:path, "Data.UDS.DiagModuleIndex"=w525:i32, "Data.UDS.UDS Control.Routine Control Identifier"=w524:u16, "Data.UDS.UDS Control.UDS RoutineControl Data"=w523:u8[])
        n200 = call "tsdiag_can_routine_control_1.vi"("data in"=w523, "mode"=w526, "ID"=w524, "ADiagModuleIndex"=w525, "path"=w527) -> ("error out"=w513:errorcluster, "success?"=w520:bool, "Return Type"=w510:i32, "path out"=w511:path, "data out"=w521:u8[])  [unwired: 2 in]
        n201 = Equal To 0?(x=w510) -> (x = 0?=w514:bool)
        n202 = call "tsapp_get_error_description.vi"("error in"=w513, "路径输入"=w511) -> ("error out"=w512:errorcluster, "ErrDes"=w515:string)  [unwired: 7 in, 1 out]
        n203 = case shown="真" w520 {
          tunnel: w528 -> [w533 w537]
          tunnel: [w532 w536] -> w522
          tunnel: w521 -> [_ w534]
          tunnel: w512 -> [w531 w535]
          frame False {
            n204 = Bundle By Name(cluster=w533, "error in"=w531) -> (w532:T3)
          }
          frame True {
            n205 = Bundle By Name(cluster=w537, "error in"=w535, "Data.UDS.UDS Control.UDS RoutineControl Read Data"=w534) -> (w536:T3)
            n206 = local write "UDS RoutineControl Read Data"(w534) -> ()
          }
        }
        n207 = Concatenate Strings("RoutineControl by Identifier fail ", w515) -> (w518:string)
        n208 = Select(t="RoutineControl by Identifier successful  ", s=w514, f=w518) -> (s? t:f=w517:string)
        n209 = call "Log.vi"("Data"=w517) -> ()  [unwired: 3 in]
      }
      frame "UDS Execute" {
        n210 = Unbundle By Name(w549) -> ("Data.Config_parameter.DLL_PATH"=w548:path, "Data.UDS.DiagModuleIndex"=w547:i32, "Data.UDS.UDS Control.Request"=w546:u8[])
        n211 = call "tstp_can_request_and_get_response.vi"("AReqDataArray"=w546, "ADiagModuleIndex"=w547, "path"=w548) -> ("错误输出"=w544:errorcluster, "Diagnostic response"=w538:u8[], "Return Type"=w543:i32, "path out"=w545:path)  [unwired: 5 in]
        "Respond" <- w538
        n212 = call "error_display.vi"("error in"=w544, "Action name"=w542, "return"=w543, "DLL path"=w545) -> ("error out"=w540:errorcluster)  [unwired: 6 in, 1 out]
        n213 = Array Size(array=w538) -> (size(s)=→"Size":i32)
        n214 = Bundle By Name(cluster=w549, "error in"=w540) -> (w541:T3)
      }
      frame "Config update" {
        n215 = Variant To Data(type=T17 {"UDS Control"={"UDS Channel Index"=0, "Request ID"=1984, "Response ID"=1992, "Request ID (Func)"=2015, "Session Mode"=1, "Reset Mode"=1, "DTC Mask"=255, "GropOfDTC"=16777215, "Seed Level"=1, "Seed"=[], "Key Level"=2, "Key"=[], "Read Identifier"=0, "UDS Read Data"=[], "ASCII Data"="", "Write Identifier"=0, "UDS Wrtie Data"=[], "IO Control Identifier"=0, "UDS IOControl Data"=[], "IO Control Mode"=0, "UDS IOControl Read Data"=[], "Routine Control Identifier"=0, "UDS RoutineControl Data"=[], "UDS RoutineControl Read Data"=[], "Routine Control Mode"=1, "SupportFDCAN"=TRUE, "time config"={"p2_timeout"=0, "p2_extended"=0, "s3_servertime"=0, "s3_clienttime"=0}, "ServiceLayer"={"FilledByte"=0, "STMin"=10, "BlockSize"=10, "FCDelay"=10, "MaxLength"=4095}, "Request"=[], "Respond"=[]}, "DiagModuleIndex"=0} ("UDS"), Variant=w559) -> (data=w553:T17, error out=w552:errorcluster)  [unwired: 1 in]
        n216 = Bundle By Name(cluster=w558, "Data.UDS"=w553, "error in"=w552) -> (w557:T3)
      }
      frame "Init" {
      }
      frame "Quit" {
        w566 = "Quit" ("y")
        n217 = local read "Create Session successful"() -> (w563:bool)
        n218 = Generate User Event(user event=w567, event data cluster=w566) -> (error out=w565:errorcluster)  [unwired: 2 in, 1 out]
        n219 = call "Log.vi"("Data"=w566) -> ()  [unwired: 3 in]
        n220 = case shown="真" w563 {
          tunnel: w565 -> [_ w574]
          tunnel: w564 -> [_ w573]
          frame False {
          }
          frame True {
            n221 = Unbundle By Name(w573) -> ("Data.Config_parameter.DLL_PATH"=w576:path, "Data.UDS.DiagModuleIndex"=w575:i32)
            n222 = call "tsdiag_can_delete.vi"("错误输入（无错误）"=w574, "ADiagModuleIndex"=w575, "path"=w576) -> ("错误输出"=w581:errorcluster, "Return Type"=w578:i32, "path out"=w580:path)  [unwired: 6 in]
            n223 = Equal To 0?(x=w578) -> (x = 0?=w577:bool)
            n224 = call "tsapp_get_error_description.vi"("error in"=w581, "ACount"=w578, "路径输入"=w580) -> ("ErrDes"=w579:string)  [unwired: 6 in, 2 out]
            n225 = Concatenate Strings("Delete Session fail ", w579) -> (w584:string)
            n226 = Select(t="Delete Session successful ", s=w577, f=w584) -> (s? t:f=w582:string)
            n227 = call "Log.vi"("Data"=w582) -> ()  [unwired: 3 in]
          }
        }
        n228 = Flush Queue(queue=w570, error in (no error)=w568) -> (queue out=w571:refnum<queue>, error out=w569:errorcluster)  [unwired: 1 out]
      }
    }
    n229 = Unbundle By Name(w247) -> ("message"=w246:string)
    n230 = Unbundle By Name(w243) -> ("error in"=w242:errorcluster)
    n231 = call "error_collect.vi"("error in (no error)"=w242) -> ("error IO"=w240:errorcluster)  [unwired: 10 in]
    n232 = case shown="\"default\", 默认" w246 {
      tunnel: w253 -> [w264 w266]
      tunnel: w252 -> [w263 w265]
      tunnel: w247 -> [w262 _]
      tunnel: [w261 w266] -> w250
      tunnel: [w260 w265] -> w249
      frame "default", Default {
        n233 = Enqueue Element(queue=w264, element=w262, error in (no error)=w263) -> (queue out=w261:refnum<queue>, error out=w260:errorcluster)  [unwired: 1 in, 1 out]
      }
      frame "" {
      }
    }
    n234 = Bundle By Name(cluster=w243, "error in"=w240) -> (w241:T3)
  }
  n235 = Release Queue(queue=w20, error in (no error)=w19) -> (error out=w18:errorcluster)  [unwired: 1 in, 2 out]
  n236 = Destroy User Event(user event=w5) -> (error out=w7:errorcluster)  [unwired: 1 in]
  n237 = Bundle By Name(cluster=w4, "Communication message"=w1) -> (→"Data out":T3)
  n238 = property class="App"(error in=w18) -> (error out=w17:errorcluster, "App.Kind"=w16:T22)  [unwired: 1 in, 1 out]
  n239 = Unregister For Events(event registration refnum=w8, error in=w7) -> ()  [unwired: 1 out]
  n240 = case shown="\"Run Time System\"" w16 {
    tunnel: w17 -> [_ _ w586 _ _ _ _]
    frame "invalid app kind", Default {
    }
    frame "Development System" {
    }
    frame "Run Time System" {
      n241 = invoke class="VI" method="FP.Close"(error in=w586) -> ()  [unwired: 2 in, 3 out]
    }
    frame "Student Edition" {
    }
    frame "Embedded LabVIEW" {
    }
    frame "Evaluation" {
    }
    frame "Custom" {
    }
  }
